vi "4Pi Capture Manager.vi"(7 "Calling VI Ref":refnum<vi>) -> ()   [LabVIEW 2016]
uses:
  4Pi Capture Manager Controls/4Pi Capture Switch Laser.ctl
  4Pi Capture Manager Controls/4Pi Capture Switch Line Scan Modes.ctl
  4Pi Capture Manager Controls/4Pi Capture Line Scan Settings.ctl
  4Pi Capture Manager Controls/DM scan mode.ctl
  <vilib>/Utility/miscctls.llb/LVPointTypeDef.ctl
  4Pi Capture Manager Controls/4Pi Capture Notifier Type.ctl
  4Pi Capture Manager Controls/4Pi Capture Actions.ctl
  4Pi Dual DM Control/4Pi Dual DM - Controls/4Pi Dual DM - Mirror Modes.ctl
  <vilib>/vision/Image Controls.llb/IMAQ Image.ctl
  Hardware Configuration/Hardware Configuration Controls/Device Type.ctl
  Hardware Configuration/Hardware Configuration Controls/Device Function.ctl
  Device Library/Cameras/Hamamatsu/Orca Flash/Orca Flash Controls/Orca Flash Actions.ctl
  Device Library/Cameras/Hamamatsu/Orca Flash/Orca Flash Controls/Orca Flash Parameters.ctl
  Device Library/Cameras/Hamamatsu/Orca Flash/Orca Flash Controls/Orca Flash Parameter List.ctl
  Device Library/Cameras/Hamamatsu/Orca Flash/Orca Flash Controls/Orca Flash ROI.ctl
  4Pi Capture Manager Controls/4Pi Capture Scan Tracker.ctl
  Device Manager/Common Device Queue/Common Device Controls/Common Device Actions.ctl
  Device Library/DAQmx/AO Single Channel Triggered Ramp/AO SCTR Type Defs/AO SCTR Actions.ctl
  Wide Field Drift Correction/WFDC Controls/WFDC External Sync.ctl
  Wide Field Drift Correction/WFDC Controls/WFDC Cycle Pause.ctl
  Wide Field Drift Correction/WFDC Controls/WFDC Status.ctl
  4Pi Dual DM Control/4Pi Dual DM - Controls/4Pi Dual DM - Standard Action.ctl
  Device Library/Stages/Stages Controls/Stage Actions.ctl
  Device Library/Shutters/Shutter Controls/Shutter Actions.ctl
  Device Library/AOTFs/AOTF Controls/AOTF Actions.ctl
  Device Library/Cameras/Camera Controls/Camera IMAQ Key Info.ctl
  Device Library/Cameras/Hamamatsu/Orca Flash/Orca Flash Controls/Orca Flash Notifier Element.ctl
  <vilib>/Utility/file.llb/Read Delimited Spreadsheet (DBL).vi
  <vilib>/Utility/file.llb/Write Delimited Spreadsheet (DBL).vi
  shell32.dll
panel:
  in  "Main Tab":T1(tab)
  in  "Sampling Time (s)":dbl min=0.0 format="%#_2f"
  out "Frame":u32(slide) scale=0.0..10.0
  out "Cycle":sgl(slide) scale=0.0..1.0
  in  "Base Save Path":path
  in  "Capture":bool
  in  "Live Preview":bool
  in  "Auto Shutter":bool=TRUE
  out "Z Step":sgl(slide) scale=0.0..1.0
  in  "File Name":string="Test Image"
  in  "Preview Exposure Time (s)":dbl=0.1 caption="Exposure Time (s)"
  in  "Capture Exposure Time (s)":dbl=0.1 caption="Exposure Time (s)"
  in  "No. of Frames":u32=1 min=1
  in  "No. of Cycles":u16=1 min=1
  in  "No. of Z Steps":u16=1 min=1
  in  "Z Step Size (µm)":dbl min=-10.0 max=10.0
  in  "Switch Laser At":T2=enum."Each Cycle"
  out "Current Cycle":u16
  out "Current Step":u16
  out "Current Frame":u32
  in  "Auto Update Subfolder":bool=TRUE
  in  "Subfolder Name":string="Area"
  in  "Current Laser":u16(ring) items=["560", "642", "405", "488", "940"]
  in  "Save As Preset":bool
  in  "Line Scan Active":bool
  in  "Number of Lines":u32=8 min=1 max=200 step=1
  in  "Line Scan Mode":T3
  in  "Line Scanning Presets":u16(ring) items=["01 FPS", "02 FPS", "04 FPS", "08 FPS", "16 FPS", "40 FPS"]
  in  "Line Scan Settings":T4
  in  "Soft trigger":bool
  in  "DM first":bool
  in  "Amp magnitude":dbl
  in  "DM scan mode":T5 items=["Idle", "Orthogonal", "Random"]
  in  "Amp step size":dbl
  in  "No. Amp steps":u16=1 min=1
  in  "Mirror Mode":u16[](array[numeric])=[1] min=1 max=140
  in  "Camera Settings":bool
  in  "Quadrants On/Off":bool
  in  "Quit":bool
  # "Live Preview"
  # "Capture"
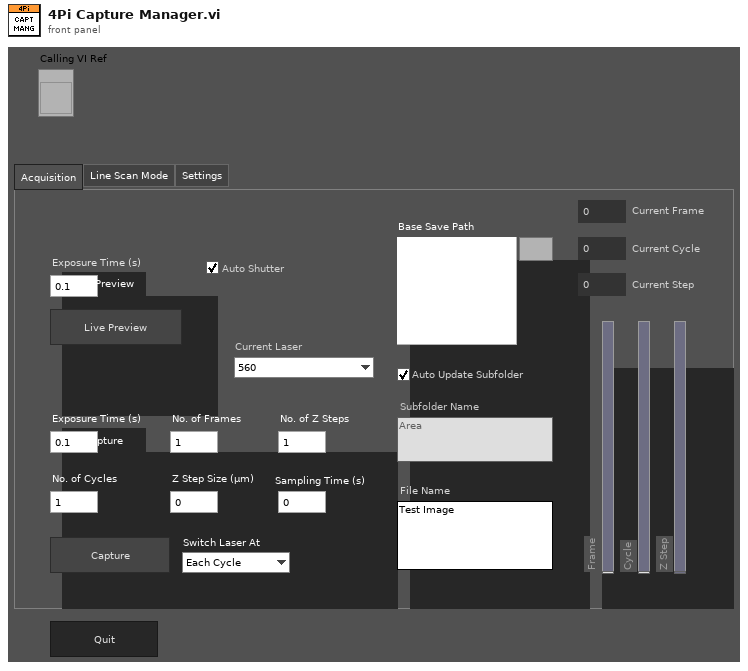
[diagram p1: front panel]
types:
  T1 = enum32{"Acquisition", "Line Scan Mode", "Settings"}
  T2 = typedef "4Pi Capture Switch Laser.ctl" = enum16{"Each Step", "Each Cycle", "All Cycles"}
  T3 = typedef "4Pi Capture Switch Line Scan Modes.ctl" = enum32{"Automatic", "Use Presets", "Manual"}
  T4 = typedef "4Pi Capture Line Scan Settings.ctl" = cluster{"Interline Interval":dbl, "Offset (V)":dbl, "Amplitude (V)":dbl, "Samples Per Channel":dbl, "Delay (ms)":dbl}
  T5 = typedef "DM scan mode.ctl" = u16
  T6 = typedef "IMAQ Image.ctl" = refnum<image>
  T7 = cluster{"Image Ref":T6, "Cycle Number":u16, "Camera Running?":bool, "Capture?":bool}
  T8 = enum8{"Enabled", "Disabled", "Disabled and Grayed Out"}
  T9 = typedef "Device Type.ctl" = enum16{"AOTF", "Camera", "Deformable Mirror", "Laser", "Flip Mirror", "Shutter", "Stage", "Waveform", "FPGA", "Email"}
  T10 = typedef "4Pi Capture Notifier Type.ctl" = cluster{"Actions":T11, "Running?":bool, "Preview Exposure (s)":dbl, "Capture Exposure (s)":dbl, "Cycles":u16, "Frames":u32, "No. of Z Steps":u16, "Z Step Size (µm)":dbl, "Base Path":path, "Init Z Position (µm)":dbl, "Lasers Lines":string[], "Save Path":path, "Line Scan?":bool, "Line Scan Mode":T3, "No. Amp steps":u16, "Amp step size":dbl, "No. Mirror Mode":u16, "DM scan mode":T5, "Metadata File Ref":refnum<file>[], "Init Mirror Modes":T12, "Sampling Time (s)":dbl}
  T11 = typedef "4Pi Capture Actions.ctl" = enum16{"Idle", "Live Preview", "Capture", "Laser On", "Laser Off", "Open Shutters", "Close Shutters", "Set Exposure Time", "Start Acquisition", "Update SubFolder", "Setup", "Camera Soft Trigger", "Camera", "Swtich1", "Switch", "Step", "Cycle", "Write DM", "External Cycle Sync", "Write Metadata", "Abort", "Quit"}
  T12 = typedef "4Pi Dual DM - Mirror Modes.ctl" = cluster{"Mode":string, "Amplitude":dbl}[]
  T13 = enum16{"Always On", "Always Off", "Off While Running"}
  T14 = typedef "LVPointTypeDef.ctl" = cluster{"Horizontal":i16, "Vertical":i16}
  T15 = typedef "Image Type" = u32
  T16 = typedef "Device Function.ctl" = enum16{"Primary", "Secondary", "Overview", "Wide Field Drift Correction", "642 nm Excitation", "560 nm Excitation", "940 nm Excitation", "546 nm Excitation", "488 nm Excitation", "405 nm Excitation", "Objective Drift Correction", "4Pi Focus Lock", "4Pi Objective Lock", "Objective XY", "Objective Z", "Sample XY", "Sample Coarse Z", "Sample Z", "4Pi Lower", "4Pi Upper", "Em Small", "Em Large", "Ex Small", "Ex Large", "Mojo", "Adj Cavity", "Line Scanning", "Alert"}
  T17 = typedef "Orca Flash Parameters.ctl" = cluster{"Value":dbl, "Parameter":T18}
  T18 = typedef "Orca Flash Parameter List.ctl" = u32
  T19 = enum32{"Page Enabled", "Page Disabled", "Page Disabled & Grayed"}
  T20 = typedef "Orca Flash ROI.ctl" = cluster{"H Offset":i32, "V Offset":i32, "H Width":i32, "V Width":i32}
  T21 = typedef "Orca Flash Actions.ctl" = enum16{"IDLE", "PREVIEW", "RECORD", "Send Trigger", "SOFT TRIGGER", "Record Settings", "SETPARAM", "GETPARAM", "SETROI", "GETROI", "PROGRESSIVE MODE", "AREA MODE", "STATUS", "QUIT"}
  T22 = typedef "4Pi Capture Scan Tracker.ctl" = cluster{"Current Step":u16, "Current Cycle":u16, "Current Laser":u16, "# of Lasers":u16, "# of Cycles":u16, "# of Steps":u16, "Switch Laser At":T2, "Current Mirror Mode":u16, "# of Mirror Mode":u16, "Current Amp step":u16, "# of Amp steps":u16}
  T23 = typedef "WFDC Status.ctl" = enum16{"Idle", "Busy", "DC Active", "Error"}
  T24 = typedef "WFDC External Sync.ctl" = cluster{"Cycle Sync":T25, "Z Offset":dbl, "WFDC Status":T23}
  T25 = typedef "WFDC Cycle Pause.ctl" = enum16{"Pause Requested", "Paused", "Resume Requested", "Resumed"}
  T26 = typedef "4Pi Dual DM - Standard Action.ctl" = enum16{"Read", "Write"}
  T27 = typedef "Stage Actions.ctl" = enum16{"Get Position", "SERVO OFF", "SERVO ON", "SERVO ON/OFF", "MVR", "MOVE", "HALT", "ONTARGET", "ERROR", "REFERENCE", "INIT", "VELOCITY", "STATUS", "EXIT", "HOME", "ZEROPOS", "NANOPOS", "ANALOG", "QUIT"}
  T28 = typedef "Shutter Actions.ctl" = enum16{"Open", "Close", "Toggle", "Status", "Quit"}
  T29 = typedef "AOTF Actions.ctl" = enum16{"Error Check", "Blank", "Line On/Off", "Set Power", "Status", "Quit"}
  T30 = typedef "AO SCTR Actions.ctl" = enum16{"Stop at Offset", "Update and Run", "Quit"}
  T31 = enum16{"open", "replace", "create", "open or create", "replace or create", "replace or create with confirmation"}
  T32 = typedef "Camera IMAQ Key Info.ctl" = cluster{"Frame":u32, "Sensor Height":i32, "Sensor Width":i32, "ROI Height":i32, "ROI Width":i32, "ROI Enable?":bool, "Bit per Pixel":u8}
  T33 = typedef "Orca Flash Notifier Element.ctl" = cluster{"Camera Actions":T21, "Received?":bool, "Running?":bool, "sCMOS Parameter":T17, "sCMOS ROI":T20, "Save Path":path, "# of frames":u32, "Image Ref":T6, "Trigger?":bool}
  T34 = typedef "Common Device Actions.ctl" = enum16{"Specific Action", "Open Front Panel", "Close Front Panel", "Quit", "Quit All"}
  T35 = typedef "4Pi Dual DM - Mirror Modes DUAL.ctl" = cluster{"Mode":string, "Amplitude":dbl}[][]
  T36 = typedef "LVRectTypeDef.ctl" = cluster{"Left":i16, "Top":i16, "Right":i16, "Bottom":i16}
  T37 = typedef "LVBoundsTypeDef.ctl" = cluster{"Width":u32, "Height":u32}
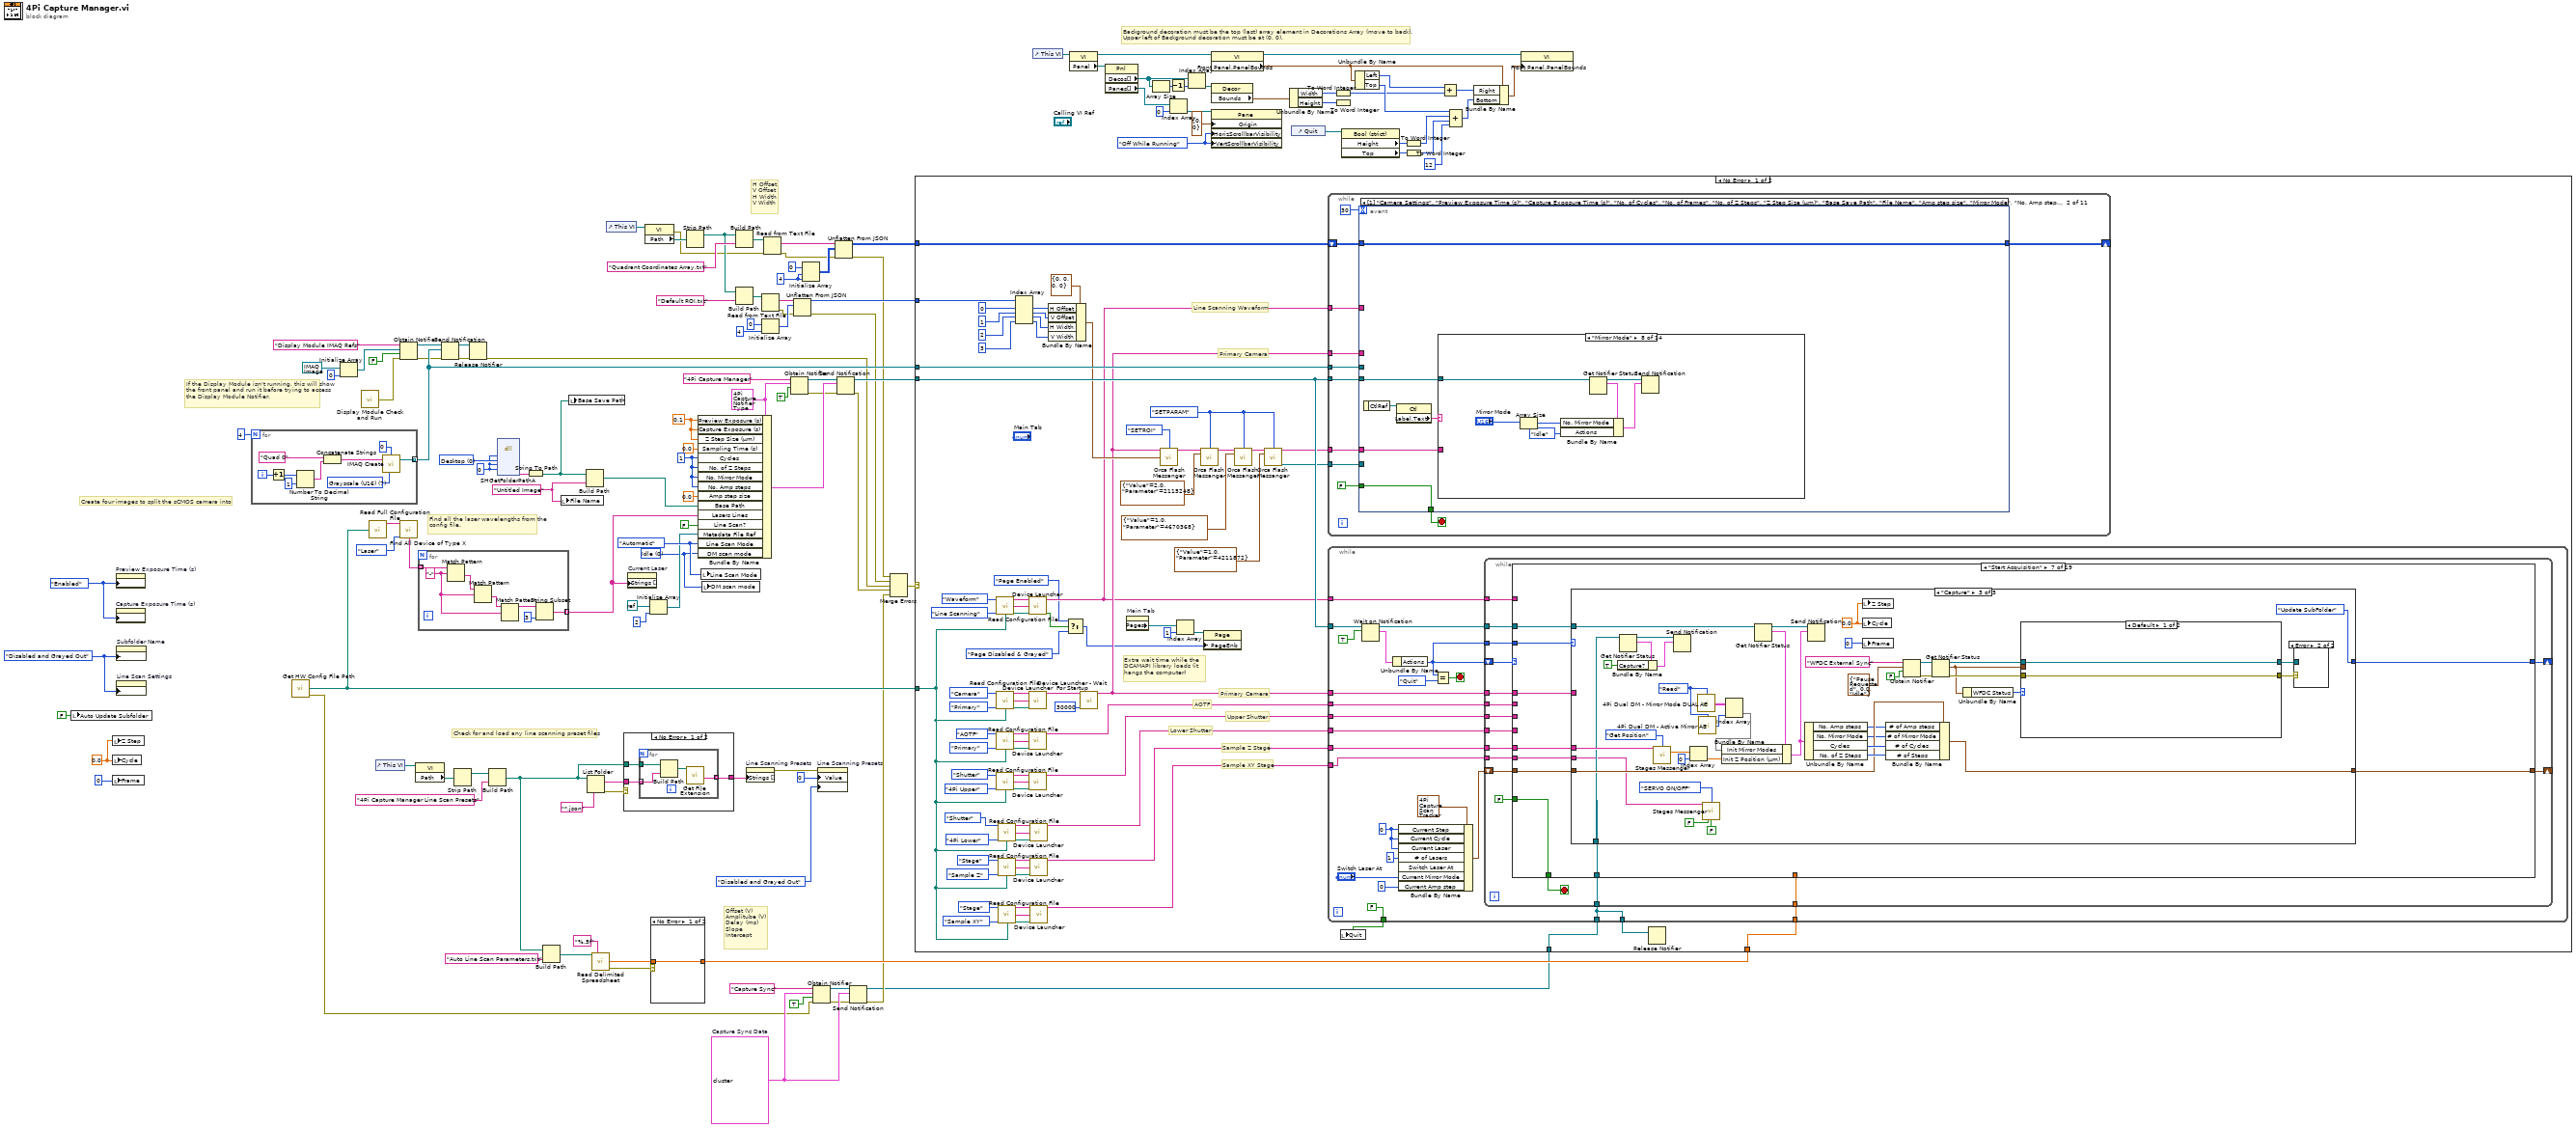
[diagram p0: block diagram]
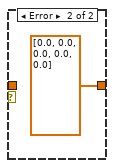
[diagram p2: hidden frame]
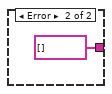
[diagram p3: hidden frame]
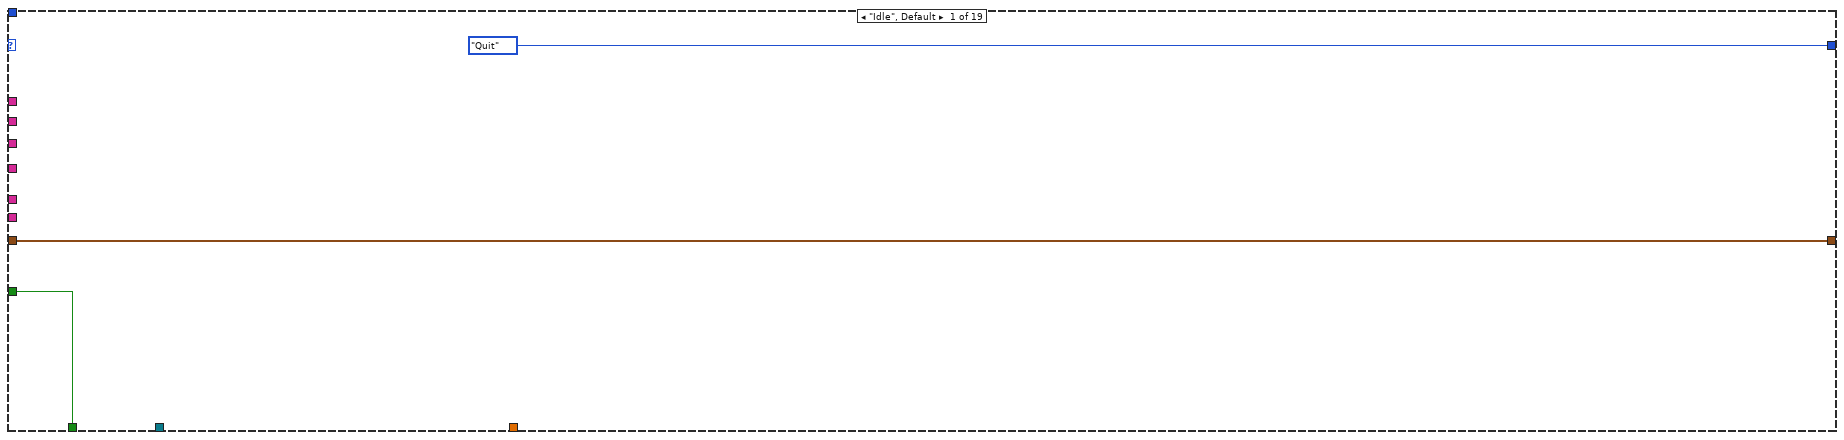
[diagram p4: hidden frame]
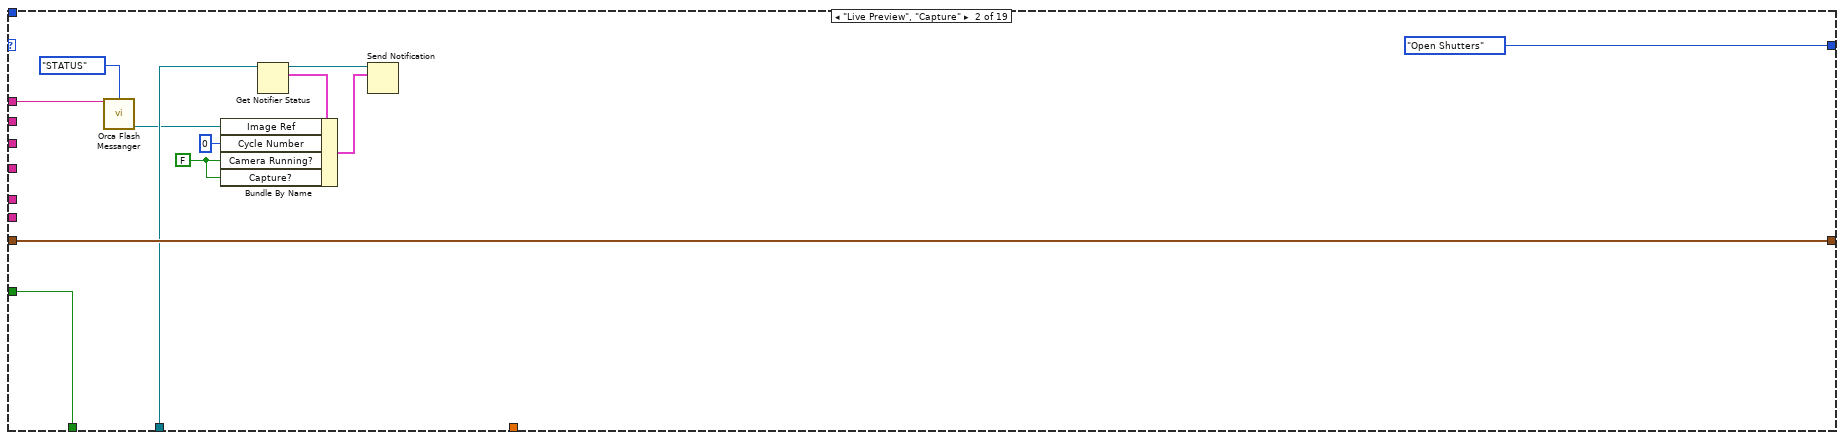
[diagram p5: hidden frame]
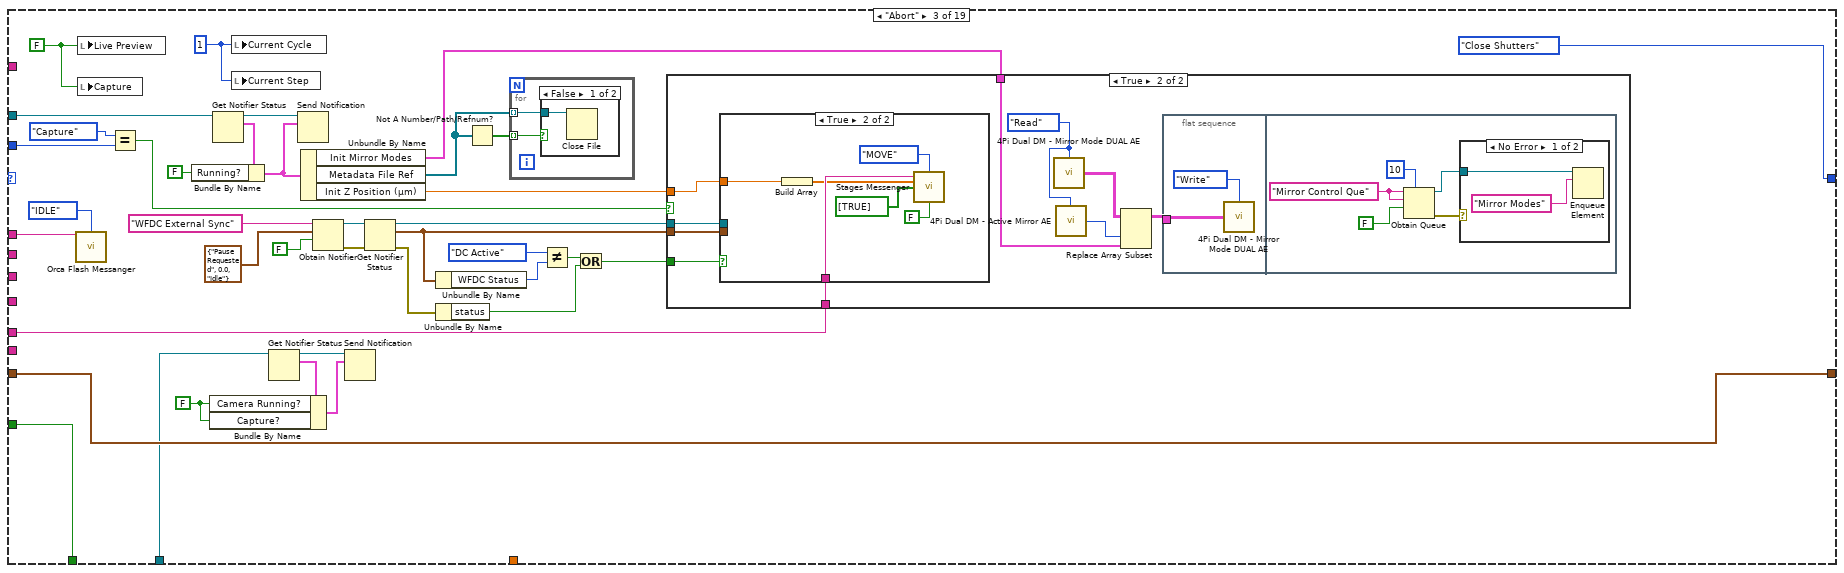
[diagram p6: hidden frame]
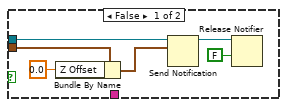
[diagram p10: hidden frame]
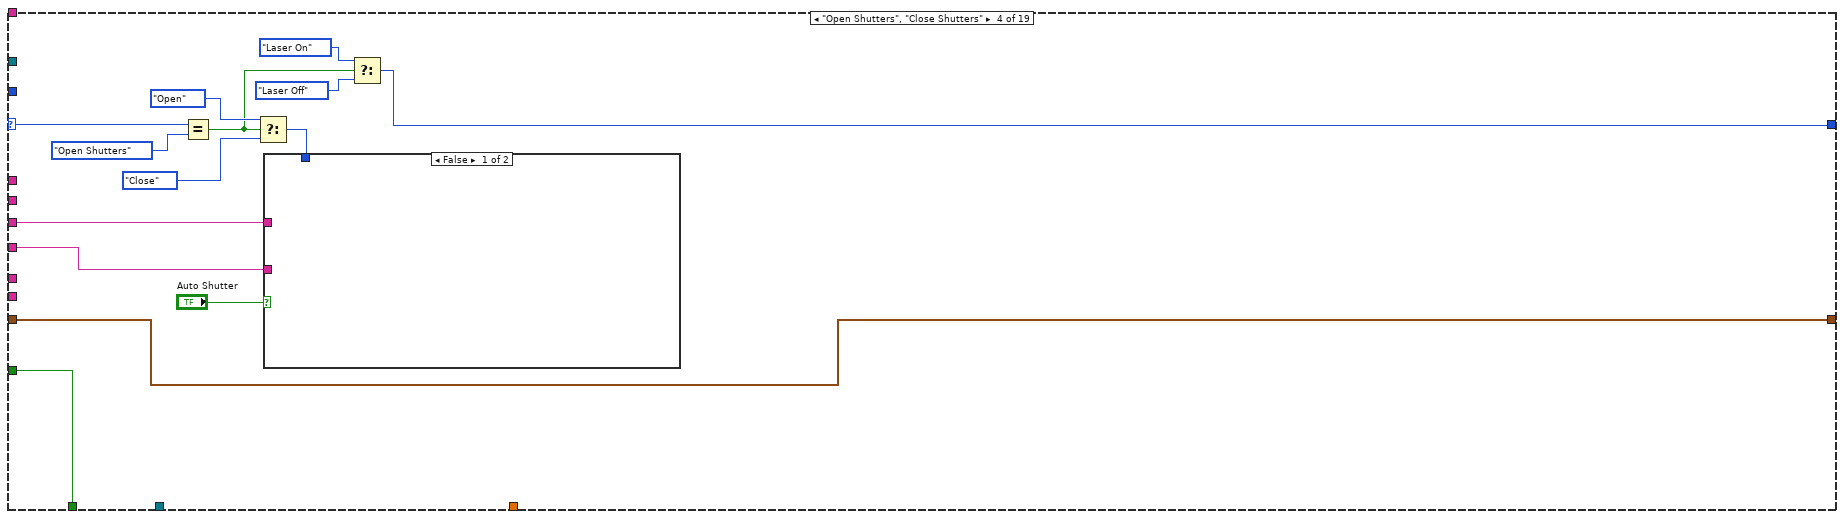
[diagram p11: hidden frame]
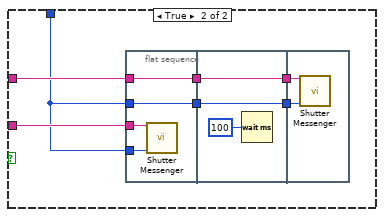
[diagram p12: hidden frame]
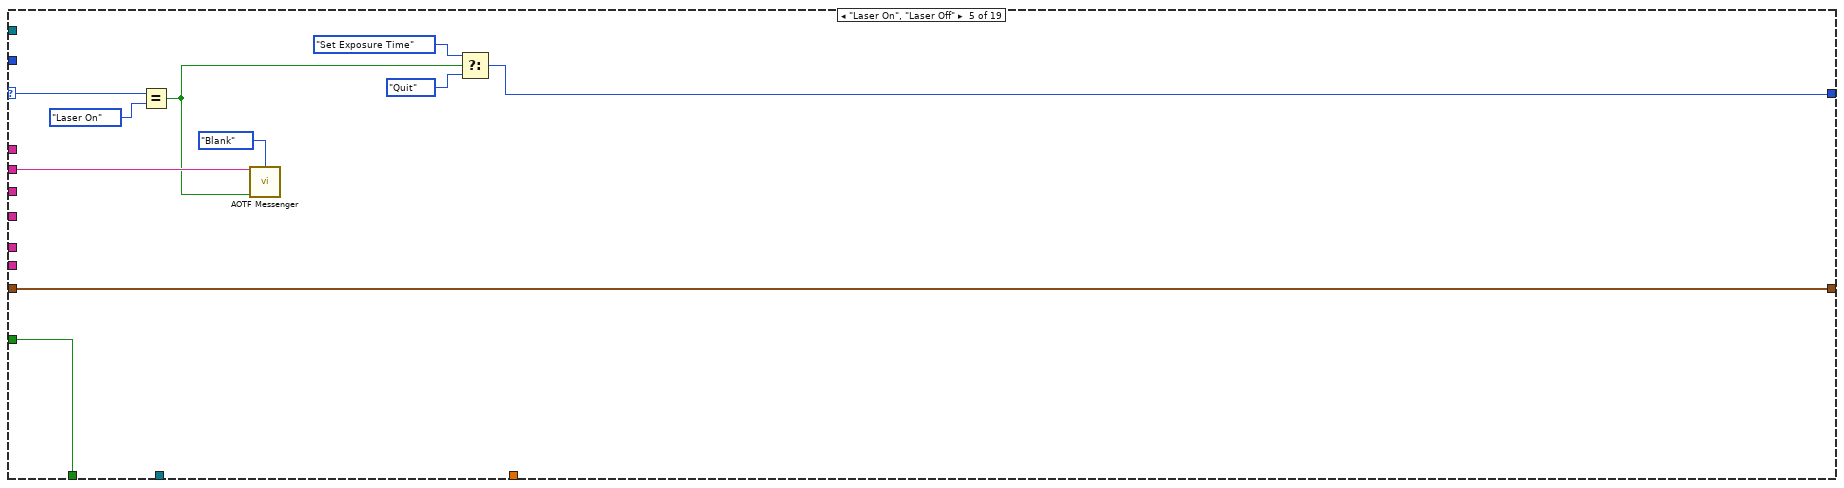
[diagram p13: hidden frame]
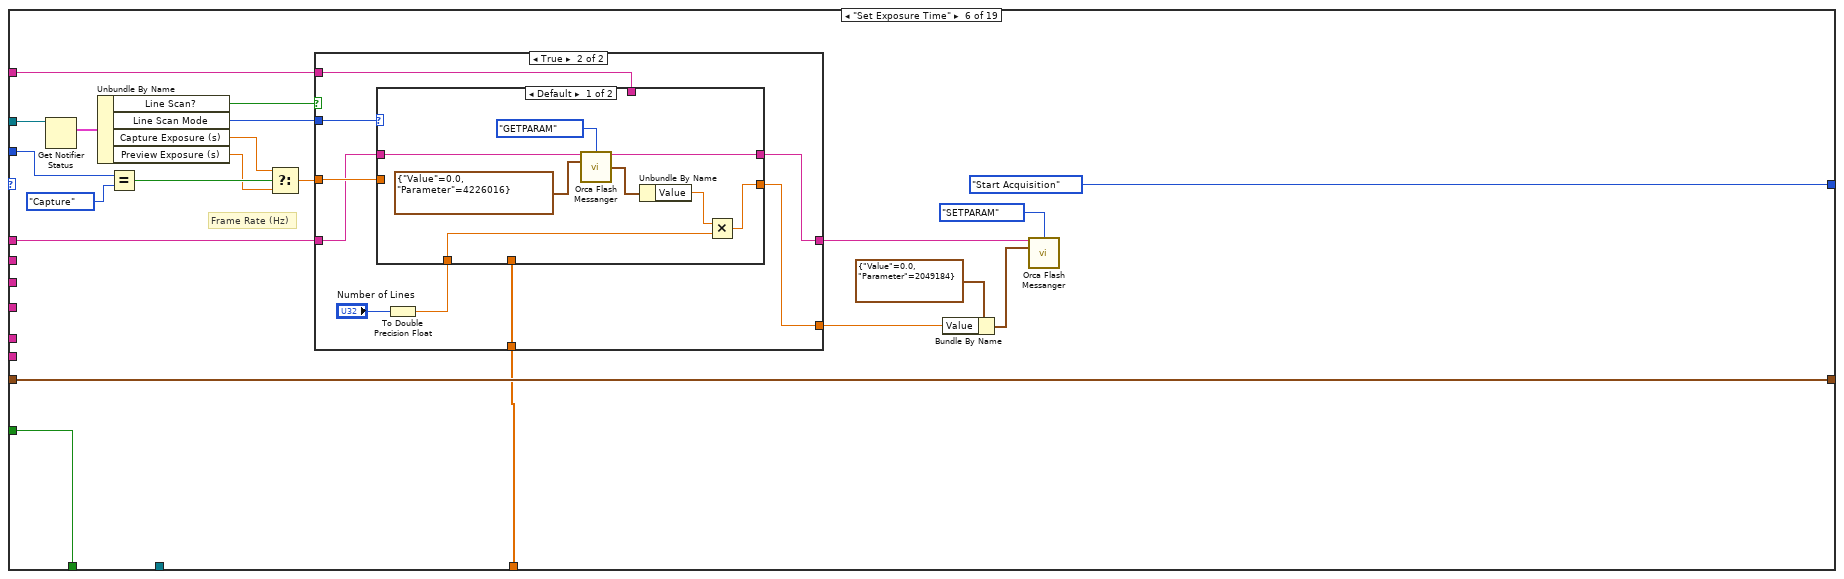
[diagram p14: hidden frame]
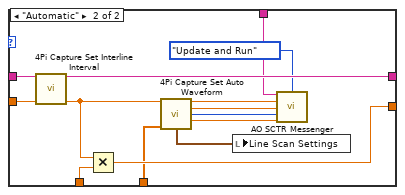
[diagram p16: hidden frame]
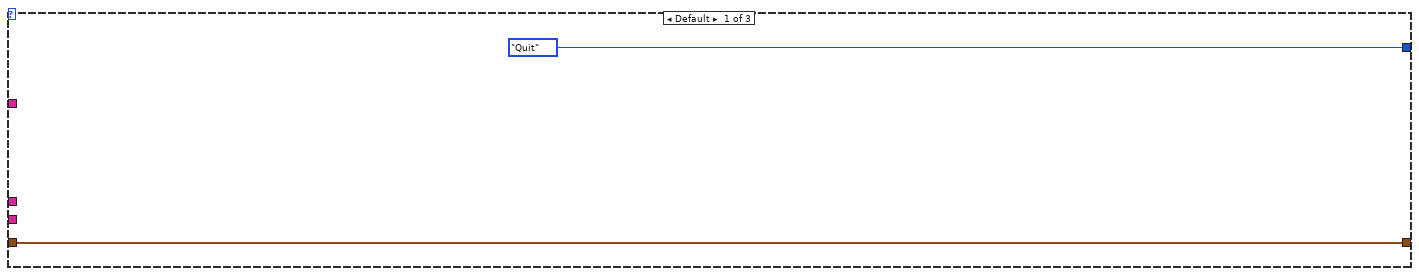
[diagram p17: hidden frame]
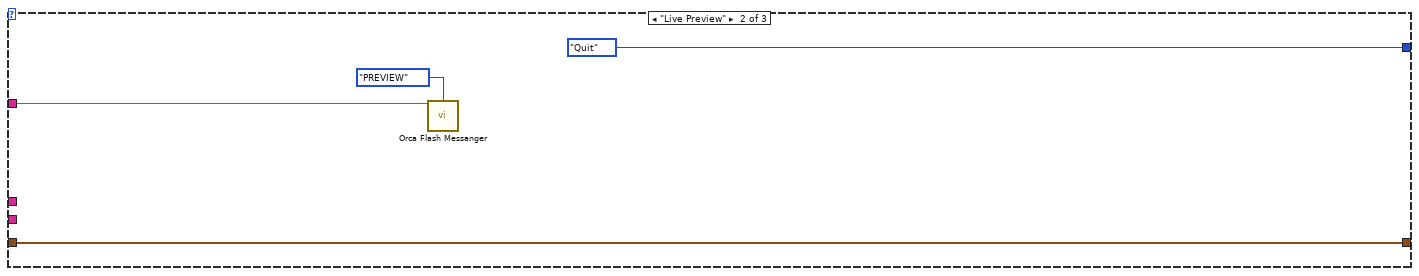
[diagram p18: hidden frame]
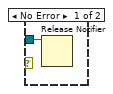
[diagram p19: hidden frame]
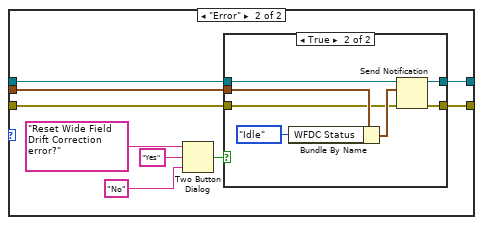
[diagram p20: hidden frame]
diagram:
  w5 = T5 0 items=["Idle", "Orthogonal", "Random"] ("DM scan mode")
  w15 = sgl 0.0 ("Cycle")
  w16 = T7 {"Image Ref"=refnum, "Cycle Number"=0, "Camera Running?"=FALSE, "Capture?"=FALSE}  # Capture Sync Data
  w28 = T8."Enabled" ("Disabled")
  w9 = 4Pi_Capture_Switch_Line_Scan_Modes."Automatic" ("Line Scan Mode")
  w29 = T8."Disabled and Grayed Out" ("Disabled")
  w76 = 4 ("dimension size")
  w80 = "Untitled Image"
  w83 = 0 items=["Desktop"=0, "Personal Documents"=5, "AppData"=26, "Local AppData"=28, "Common AppData"=35, "Program Files"=38, "Program Files Common"=43, "Common Documents"=46] ("Requested Path")
  w82 = 0 ("HWND")
  w4 = u16 1 ("Cycles")
  w3 = 0.1 ("Preview Exposure (s)")
  w86 = T10 {"Actions"=enum."Live Preview", "Running?"=FALSE, "Preview Exposure (s)"=0.1, "Capture Exposure (s)"=0.1, "Cycles"=1, "Frames"=0, "No. of Z Steps"=0, "Z Step Size (µm)"=0.0, "Base Path"=path "", "Init Z Position (µm)"=0.0, "Lasers Lines"=[], "Save Path"=path "", "Line Scan?"=FALSE, "Line Scan Mode"=enum."Automatic", "No. Amp steps"=0, "Amp step size"=0.0, "No. Mirror Mode"=0, "DM scan mode"=0, "Metadata File Ref"=[], "Init Mirror Modes"=[], "Sampling Time (s)"=0.0} ("4Pi Capture Notifier Type")
  w108 = T13."Off While Running" ("Vertical Scrollbar Visibility")
  # "Offset (V)\nAmplitube (V)\nDelay (ms)\nSlope\nIntercept"
  # "Check for and load any line scanning preset files"
  # "Find all the laser wavelengths from the config file."
  # "If the Display Module isn't running, this will show the front panel and run it before trying to access the Display Module Notifier."
  # "H Offset\nV Offset\nH Width\nV Width"
  # "Create four images to split the sCMOS camera into"
  # "Background decoration must be the top (last) array element in Decorations Array (move to back).\nUpper left of Background decoration must be at (0, 0)."
  n1 = local write "Auto Update Subfolder"(FALSE ("Auto Update Subfolder")) -> ()
  n2 = local write "Z Step"(w15) -> ()
  n3 = local write "Cycle"(w15) -> ()
  n4 = local write "Frame"(u32 0 ("Frame")) -> ()
  n5 = property on="Preview Exposure Time (s)" class="DigNum (strict)"("DisabledEnum"=w28) -> ()  [unwired: 2 in, 2 out]
  n6 = property on="Capture Exposure Time (s)" class="DigNum (strict)"("DisabledEnum"=w28) -> ()  [unwired: 2 in, 2 out]
  n7 = property on="Subfolder Name" class="Str"("DisabledEnum"=w29) -> ()  [unwired: 2 in, 2 out]
  n8 = property on="Line Scan Settings" class="Clust (strict)"("DisabledEnum"=w29) -> ()  [unwired: 2 in, 2 out]
  n9 = for {
    N: 4 -> [_]
    tunnel: [w126] -> w90 mode=indexing
    i -> [w134]
    w129 = T15 7 items=["Grayscale (U8)", "Grayscale (I16)", "Grayscale (SGL)", "Complex (CSG)", "RGB (U32)", "HSL (U32)", "RGB (U64)", "Grayscale (U16)"] ("Image Type")
    n10 = Increment(x=w134) -> (x+1=w132:i32)
    n11 = Number To Decimal String(number=w132, width (-)=i16 1) -> (decimal integer string=w130:string)
    n12 = Concatenate Strings("Quad 0" ("name (unnamed)"), w130) -> (w127:string)
    n13 = call "IMAQ Create"("Border Size"=0, "Image Name"=w127, "Image Type"=w129) -> ("New Image"=w126:T6)  [unwired: 2 in, 1 out]
  }
  n14 = call "Get HW Config File Path.vi"() -> ("File Path"=w43:path, "Error"=w13:errorcluster)  [unwired: 14 in]
  n15 = Initialize Array(T6 refnum ("New Image"), 0 ("dimension size")) -> (w48:T6[])
  n16 = call "Display Module Check and Run.vi"() -> ("Error"=w47:errorcluster)  [unwired: 15 in]
  n17 = call "Read Full Configuration File.vi"("Config File Path"=w43) -> ("Unique Notifier Names"=w44:string[])  [unwired: 11 in, 3 out]
  n18 = control-ref of="This VI"() -> (w40:refnum<vi>)
  n19 = Obtain Notifier(name (unnamed)="Display Module IMAQ Refs", notification data type=w48, create if not found? (T)=FALSE, error in (no error)=w47) -> (notifier out=w91:refnum<notifier>, error out=w58:errorcluster)  [unwired: 1 out]
  n20 = call "Find All Device of Type X.vi"("Unique Notifier Names"=w44, "Device Type"=Device_Type."Laser") -> ("All Devices"=w46:string[])  [unwired: 12 in, 1 out]
  n21 = property class="VI"(reference=w40) -> ("Path"=w39:path)  [unwired: 1 in, 2 out]
  n22 = for {
    tunnel: w46 -> [w136] mode=indexing
    tunnel: [w135] -> w20 mode=indexing
    w139 = "-" ("regular expression")
    n23 = Match Pattern(string=w136, regular expression=w139) -> (after substring=w137:string)  [unwired: 1 in, 3 out]
    n24 = Match Pattern(string=w137, regular expression=w139) -> (after substring=w138:string)  [unwired: 1 in, 3 out]
    n25 = Match Pattern(string=w138, regular expression=w139) -> (before substring=w140:string)  [unwired: 1 in, 3 out]
    n26 = String Subset(string=w140, length (rest)=3 ("length (rest)")) -> (substring=w135:string)  [unwired: 1 in]
  }
  n27 = Send Notification(notification=w90, notifier=w91, error in (no error)=w58) -> (notifier out=w78:refnum<notifier>, error out=w63:errorcluster)
  n28 = Strip Path(path=w39) -> (stripped path=w38:path)  [unwired: 1 out]
  n29 = Release Notifier(notifier=w78, error in (no error)=w63) -> (error out=w55:errorcluster)  [unwired: 1 in, 2 out]
  n30 = Build Path(base path=w38, name or relative path="4Pi Capture Manager Line Scan Presets") -> (appended path=w27:path)
  n31 = dll-call lib="shell32.dll" fn="SHGetFolderPathA"("HWND"=w82, "nFolder"=w83, "hToken"=w82, "dwFlags"=w82) -> ("pszPath"=w81:string)  [unwired: 9 in, 2 out]
  n32 = String To Path(string=w81) -> (path=w79:path)
  n33 = Build Path(base path=w27, name or relative path="Auto Line Scan Parameters.txt") -> (appended path=w25:path)
  n34 = local write "File Name"(w80) -> ()
  n35 = local write "Base Save Path"(w79) -> ()
  n36 = Build Path(base path=w79, name or relative path=w80) -> (appended path=w84:path)
  n37 = List Folder(path=w27, pattern="*.json") -> (filenames=w35:string[], error out=w34:errorcluster)  [unwired: 2 in, 2 out]
  n38 = call-poly <vilib>:"Read Delimited Spreadsheet.vi"("file path (dialog if empty)"=w25, "format (%.3f)"="%.5f") -> ("first row"=w22:dbl[], "error out"=w23:errorcluster)  [unwired: 8 in, 4 out]
  n39 = control-ref of="This VI"() -> (w89:refnum<vi>)
  n40 = case shown="No Error" w34 {
    tunnel: w35 -> [w144 _]
    tunnel: w27 -> [w143 _]
    tunnel: [w142 string[] []] -> w33
    frame No Error {
      n41 = for {
        tunnel: w144 -> [w147] mode=indexing
        tunnel: w143 -> [w148]
        tunnel: [w145] -> w142 mode=indexing
        n42 = Build Path(base path=w148, name or relative path=w147) -> (appended path=w146:path)
        n43 = call <vilib>:"Get File Extension.vi"("file"=w146) -> ("filename without extension"=w145:string)  [unwired: 6 in, 4 out]
      }
    }
    frame Error {
    }
  }
  n44 = property on="Current Laser" class="Ring (strict)"("Strings []"=w20) -> ()  [unwired: 2 in, 2 out]
  n45 = property class="VI"(reference=w89) -> (error out=w60:errorcluster, "Path"=w88:path)  [unwired: 1 in, 1 out]
  n46 = Initialize Array(refnum<k0> refnum, 2 ("dimension size")) -> (w6:refnum<k0>[])
  n47 = case shown="No Error" w23 {
    tunnel: w22 -> [w150 _]
    tunnel: [w150 dbl[] [0.0, 0.0, 0.0, 0.0, 0.0] ("first row")] -> w21
    frame No Error {
    }
    frame Error {
    }
  }
  n48 = Strip Path(path=w88) -> (stripped path=w71:path)  [unwired: 1 out]
  n49 = Bundle By Name(cluster=w86, "Preview Exposure (s)"=w3, "Capture Exposure (s)"=w3, "Z Step Size (µm)"=w3, "Sampling Time (s)"=0.0, "Cycles"=w4, "No. of Z Steps"=w4, "No. Mirror Mode"=w4, "No. Amp steps"=w4, "Amp step size"=0.0, "Base Path"=w84, "Lasers Lines"=w20, "Line Scan?"=FALSE, "Metadata File Ref"=w6, "Line Scan Mode"=w9, "DM scan mode"=w5) -> (w85:T10)
  n50 = local write "Line Scan Mode"(w9) -> ()
  n51 = local write "DM scan mode"(w5) -> ()
  n52 = Build Path(base path=w71, name or relative path="Quadrant Coordinates Array.txt") -> (appended path=w74:path)
  n53 = Build Path(base path=w71, name or relative path="Default ROI.txt") -> (appended path=w69:path)
  n54 = property on="Line Scanning Presets" class="Ring (strict)"("Strings []"=w33) -> (error out=w32:errorcluster)  [unwired: 2 in, 1 out]
  n55 = Read from Text File(file (use dialog)=w69) -> (text=w68:string, error out=w61:errorcluster)  [unwired: 3 in, 2 out]
  n56 = Initialize Array(0 ("element"), 4 ("dimension size")) -> (w65:i32[])
  n57 = Read from Text File(file (use dialog)=w74, error in=w60) -> (text=w73:string, error out=w59:errorcluster)  [unwired: 2 in, 2 out]
  n58 = Obtain Notifier(name (unnamed)="4Pi Capture Manager", notification data type=w86, create if not found? (T)=TRUE) -> (notifier out=w94:refnum<notifier>, error out=w62:errorcluster)  [unwired: 1 in, 1 out]
  n59 = Unflatten From JSON(JSON string=w68, type and defaults=w65, error in (no error)=w61) -> (value=w64:i32[], error out=w54:errorcluster)  [unwired: 4 in]
  n60 = Initialize Array(0 ("element"), w76, w76) -> (w75:i32[][])
  n61 = Obtain Notifier(name (unnamed)="Capture Sync", notification data type=w16, create if not found? (T)=TRUE, error in (no error)=w13) -> (notifier out=w17:refnum<notifier>, error out=w12:errorcluster)  [unwired: 1 out]
  n62 = property on="Line Scanning Presets" class="Ring (strict)"(error in=w32, "Value"=u16 0, "DisabledEnum"=T8."Disabled and Grayed Out" ("Disabled")) -> ()  [unwired: 1 in, 2 out]
  n63 = Unflatten From JSON(JSON string=w73, type and defaults=w75, error in (no error)=w59) -> (value=w72:i32[][], error out=w53:errorcluster)  [unwired: 4 in]
  n64 = Send Notification(notification=w85, notifier=w94, error in (no error)=w62) -> (notifier out=w93:refnum<notifier>, error out=w56:errorcluster)
  n65 = Send Notification(notification=w16, notifier=w17, error in (no error)=w12) -> (notifier out=w10:refnum<notifier>, error out=w11:errorcluster)
  n66 = Merge Errors(w53, w54, w55, w56, w11) -> (w57:errorcluster)
  n67 = case shown="No Error" w57 {
    tunnel: w43 -> [w153 _]
    tunnel: w93 -> [w211 w1561]
    tunnel: w90 -> [w199 w1559]
    tunnel: w72 -> [w198 _]
    tunnel: w64 -> [w192 _]
    tunnel: w21 -> [w173 _]
    tunnel: w10 -> [w165 _]
    frame No Error {
      w159 = Orca_Flash_Actions."SETPARAM" ("Camera Actions")
      # "Sample XY Stage"
      # "Line Scanning Waveform"
      # "Primary Camera"
      # "Extra wait time while the DCAMAPI library loads (it hangs the computer)"
      # "Sample Z Stage"
      # "Lower Shutter"
      # "Upper Shutter"
      # "AOTF"
      # "Primary Camera"
      n68 = call "Read Configuration File.vi"("Device Type"=Device_Type."Waveform", "Device Function"=Device_Function."Line Scanning", "Config File Path"=w153) -> ("Unique Notifier Name"=w177:string, "Device Ports/IDs/Channels"=w178:string[], "Device Engine Path"=w175:path)  [unwired: 9 in, 1 out]
      n69 = call "Read Configuration File.vi"("Device Type"=Device_Type."Camera", "Device Function"=Device_Function."Primary", "Config File Path"=w153) -> ("Unique Notifier Name"=w231:string, "Device Ports/IDs/Channels"=w230:string[], "Device Engine Path"=w229:path)  [unwired: 9 in, 1 out]
      n70 = call "Read Configuration File.vi"("Device Type"=Device_Type."AOTF", "Device Function"=Device_Function."Primary", "Config File Path"=w153) -> ("Unique Notifier Name"=w222:string, "Device Ports/IDs/Channels"=w223:string[], "Device Engine Path"=w224:path)  [unwired: 9 in, 1 out]
      n71 = call "Read Configuration File.vi"("Device Type"=Device_Type."Shutter", "Device Function"=Device_Function."4Pi Upper", "Config File Path"=w153) -> ("Unique Notifier Name"=w212:string, "Device Ports/IDs/Channels"=w221:string[], "Device Engine Path"=w220:path)  [unwired: 9 in, 1 out]
      n72 = call "Read Configuration File.vi"("Device Type"=Device_Type."Shutter", "Device Function"=Device_Function."4Pi Lower", "Config File Path"=w153) -> ("Unique Notifier Name"=w213:string, "Device Ports/IDs/Channels"=w216:string[], "Device Engine Path"=w217:path)  [unwired: 9 in, 1 out]
      n73 = call "Read Configuration File.vi"("Device Type"=Device_Type."Stage", "Device Function"=Device_Function."Sample Z", "Config File Path"=w153) -> ("Unique Notifier Name"=w206:string, "Device Ports/IDs/Channels"=w204:string[], "Device Engine Path"=w203:path)  [unwired: 9 in, 1 out]
      n74 = call "Read Configuration File.vi"("Device Type"=Device_Type."Stage", "Device Function"=Device_Function."Sample XY", "Config File Path"=w153) -> ("Unique Notifier Name"=w154:string, "Device Ports/IDs/Channels"=w158:string[], "Device Engine Path"=w157:path)  [unwired: 9 in, 1 out]
      n75 = Index Array(array=w192, index #1=0 ("index"), index #2=1 ("index"), index #3=2 ("index"), index #4=3 ("index")) -> (element #1=w187:i32, element #2=w184:i32, element #3=w185:i32, element #4=w186:i32)
      n76 = call "Device Launcher.vi"("Notifier Name"=w177, "Device Ports/IDs/Channels"=w178, "Device Engine Path"=w175) -> ("Notifier Name"=w174:string, "Running?"=w169:bool)  [unwired: 11 in]
      n77 = call "Device Launcher.vi"("Notifier Name"=w231, "Device Ports/IDs/Channels"=w230, "Device Engine Path"=w229) -> ("Notifier Name"=w181:string)  [unwired: 11 in, 1 out]
      n78 = call "Device Launcher.vi"("Notifier Name"=w222, "Device Ports/IDs/Channels"=w223, "Device Engine Path"=w224) -> ("Notifier Name"=w210:string)  [unwired: 11 in, 1 out]
      n79 = call "Device Launcher.vi"("Notifier Name"=w212, "Device Ports/IDs/Channels"=w221, "Device Engine Path"=w220) -> ("Notifier Name"=w209:string)  [unwired: 11 in, 1 out]
      n80 = call "Device Launcher.vi"("Notifier Name"=w213, "Device Ports/IDs/Channels"=w216, "Device Engine Path"=w217) -> ("Notifier Name"=w208:string)  [unwired: 11 in, 1 out]
      n81 = call "Device Launcher.vi"("Notifier Name"=w206, "Device Ports/IDs/Channels"=w204, "Device Engine Path"=w203) -> ("Notifier Name"=w201:string)  [unwired: 11 in, 1 out]
      n82 = call "Device Launcher.vi"("Notifier Name"=w154, "Device Ports/IDs/Channels"=w158, "Device Engine Path"=w157) -> ("Notifier Name"=w152:string)  [unwired: 11 in, 1 out]
      n83 = Bundle By Name(cluster=T20 {"H Offset"=0, "V Offset"=0, "H Width"=0, "V Width"=0} ("Orca Flash ROI"), "H Offset"=w187, "V Offset"=w184, "H Width"=w185, "V Width"=w186) -> (w183:T20)
      n84 = Select(t=T19."Page Enabled" ("Page Enabled State"), s=w169, f=T19."Page Disabled & Grayed" ("Page Enabled State")) -> (s? t:f=w166:T19)
      n85 = call "Device Launcher - Wait For Startup.vi"("Notifier Name"=w181, "Wait Time (ms)"=30000) -> ("Notifier Name (Dup)"=w180:string)  [unwired: 12 in, 1 out]
      n86 = property on="Main Tab" class="TabCtl (strict)"() -> ("Pages"=w172:refnum<vi>[])  [unwired: 2 in, 2 out]
      n87 = call "Orca Flash Messanger.vi"("Notifier Name"=w180, "Camera Actions"=Orca_Flash_Actions."SETROI", "sCMOS ROI"=w183) -> ("Notifier Name Dup"=w197:string)  [unwired: 8 in, 4 out]
      n88 = Index Array(array=w172, index=1) -> (element=w170:refnum<vi>)
      n89 = call "Orca Flash Messanger.vi"("Notifier Name"=w197, "Camera Actions"=w159, "sCMOS Parameter"=T17 {"Value"=2.0, "Parameter"=2115248}) -> ("Notifier Name Dup"=w196:string)  [unwired: 8 in, 4 out]
      n90 = property class="Page"(reference=w170, "PageEnb"=w166) -> ()  [unwired: 1 in, 2 out]
      n91 = call "Orca Flash Messanger.vi"("Notifier Name"=w196, "Camera Actions"=w159, "sCMOS Parameter"=T17 {"Value"=1.0, "Parameter"=4670368}) -> ("Notifier Name Dup"=w163:string)  [unwired: 8 in, 4 out]
      n92 = call "Orca Flash Messanger.vi"("Notifier Name"=w163, "Camera Actions"=w159, "sCMOS Parameter"=T17 {"Value"=1.0, "Parameter"=4211872}) -> ("Notifier Name Dup"=w162:string, "Image Ref"=w161:T6)  [unwired: 8 in, 3 out]
      n93 = while {
        tunnel: w211 -> [w1161]
        tunnel: w162 -> [w1160]
        tunnel: w161 -> [w1158]
        tunnel: w199 -> [w1157]
        shift-right: [w1155] -> _
        shift-left: w198 -> [w1156]
        tunnel: w180 -> [w1154]
        tunnel: w174 -> [w1153]
        stop <- w1163 stop-if-true
        n94 = event shown="[1] \"Camera Settings\", \"Preview Exposure Time (s)\", \"Capture Exposure Time (s)\", \"No. of Cycles\", \"No. of Frames\", \"No. of Z Steps\", \"Z Step Size (µm)\", \"Base Save Path\", \"File Name\", \"Amp step size\", \"Mirror Mode\", \"No. Amp steps\", \"DM scan mode\", \"Sampling Time (s)\": Value Change" {
          selector: _ -> [_ _ _ _ _ _ _ _ _ _ _]
          dyn-events: _ -> [_ _ _ _ _ _ _ _ _ _ _]
          timeout: 30 -> [_ _ _ _ _ _ _ _ _ _ _]
          tunnel: [w1187 w1225 w1344 w1365 w1421 w1446 w1468 w1484 w1504 w1528 w1557] -> w1163
          tunnel: FALSE -> [w1187 w1225 w1344 w1365 w1421 w1446 w1468 w1484 w1504 w1528 _]
          tunnel: w1161 -> [w1181 w1222 w1341 _ _ w1440 w1466 _ w1502 _ w1556]
          tunnel: w1160 -> [_ w1221 _ _ _ _ _ _ _ _ _]
          tunnel: w1158 -> [w1185 _ _ w1349 _ _ _ _ _ _ _]
          tunnel: w1157 -> [w1186 _ _ w1355 _ _ _ _ _ _ w1544]
          tunnel: w1156 -> [w1184 w1220 w1333 w1348 w1416 w1423 w1467 w1485 w1503 w1520 w1543]
          tunnel: [w1184 w1220 w1333 w1347 w1416 w1423 w1467 w1485 w1503 w1520 w1543] -> w1155
          tunnel: w1154 -> [_ _ _ _ _ w1434 _ _ w1488 _ _]
          tunnel: w1153 -> [_ _ _ _ _ w1424 _ _ w1496 _ _]
          event Timeout {
            # "Convert to array and then crop. If you\nextract or mask image the destination\nimage custom data keys are overwritten."
            n95 = event-data() -> ()  [unwired: 1 in, 1 out]
            n96 = call "IMAQ ImageToArray"("Image"=w1185) -> ("Image Pixels (U16)"=w1183:u16[][])  [unwired: 3 in, 4 out]
            n97 = for {
              tunnel: w1186 -> [w1218] mode=indexing
              tunnel: w1183 -> [w1219]
              tunnel: w1184 -> [w1216] mode=indexing
              n98 = Index Array(array=w1216, index #1=0 ("index"), index #2=2 ("index"), index #3=1 ("index"), index #4=3 ("index")) -> (element #1=w1214:i32, element #2=w1213:i32, element #3=w1209:i32, element #4=w1208:i32)
              n99 = Array Subset(array=w1219, index (row)=w1214, length (row)=w1213, index (col)=w1209, length (col)=w1208) -> (w1217:u16[][])
              n100 = call "IMAQ ArrayToImage"("Image Pixels (U16)"=w1217, "Image"=w1218) -> ()  [unwired: 8 in, 2 out]
            }
            n101 = local read "Soft trigger"() -> (w1166:bool)
            n102 = local read "No. Amp steps"() -> (w1165:u16)
            n103 = case shown="True" w1166 {
              tunnel: [w1188 w1189] -> w1164
              tunnel: w1165 -> [_ w1190]
              frame False {
                n104 = local read "No. of Frames"() -> (w1188:u32)
              }
              frame True {
                n105 = To Unsigned Long Integer(number=w1190) -> (unsigned 32bit integer=w1189:u32)
                n106 = local write "No. of Frames"(w1189) -> ()
              }
            }
            n107 = local read "Mirror Mode"() -> (w1175:u16[])
            n108 = local read "Soft trigger"() -> (w1168:bool)
            n109 = local read "DM scan mode"() -> (w1173:T5)
            n110 = local read "No. of Cycles"() -> (w1171:u16)
            n111 = local read "Amp step size"() -> (w1176:dbl)
            n112 = local read "DM first"() -> (w1169:bool)
            n113 = local read "Z Step Size (µm)"() -> (w1177:dbl)
            n114 = local read "No. of Z Steps"() -> (w1178:u16)
            n115 = Array Size(array=w1175) -> (size(s)=w1172:i32)
            n116 = Or(x=w1169, y=w1168) -> (x .or. y?=w1167:bool)
            n117 = case shown="1" w1173 {
              tunnel: w1172 -> [_ w1195]
              tunnel: w1165 -> [_ w1196]
              tunnel: [w1191 w1194] -> w1170
              tunnel: w1167 -> [_ w1193]
              tunnel: w1171 -> [w1191 w1192]
              frame Default {
              }
              frame 1 {
                n118 = case shown="True" w1193 {
                  tunnel: w1196 -> [w1202 _]
                  tunnel: w1195 -> [w1201 w1207]
                  tunnel: [w1197 w1206] -> w1194
                  tunnel: w1192 -> [_ _]
                  frame False {
                    n119 = To Unsigned Word Integer(number=w1201) -> (unsigned 16bit integer=w1200:u16)
                    n120 = Multiply(x=w1200, y=w1202) -> (x*y=w1198:u16)
                    n121 = Equal To 0?(x=w1198) -> (x = 0?=w1199:bool)
                    n122 = case shown="False" w1199 {
                      tunnel: w1198 -> [w1203 w1205]
                      tunnel: [w1203 w1204] -> w1197
                      frame False {
                      }
                      frame True {
                        n123 = Increment(x=w1205) -> (x+1=w1204:u16)
                      }
                    }
                  }
                  frame True {
                    n124 = To Unsigned Word Integer(number=w1207) -> (unsigned 16bit integer=w1206:u16)
                  }
                }
              }
            }
            n125 = Get Notifier Status(notifier=w1181) -> (notifier out=w1182:refnum<notifier>, current notification=w1180:T10)  [unwired: 1 in, 3 out]
            n126 = Bundle By Name(cluster=w1180, "Actions"=4Pi_Capture_Actions."Idle", "Frames"=w1164, "No. of Z Steps"=w1178, "Z Step Size (µm)"=w1177, "No. Amp steps"=w1165, "Amp step size"=w1176, "No. Mirror Mode"=w1172, "DM scan mode"=w1173, "Cycles"=w1170) -> (w1179:T10)
            n127 = Send Notification(notification=w1179, notifier=w1182) -> ()  [unwired: 1 in, 2 out]
            n128 = local write "No. of Cycles"(w1170) -> ()
          }
          event "Camera Settings", "Preview Exposure Time (s)", "Capture Exposure Time (s)", "No. of Cycles", "No. of Frames", "No. of Z Steps", "Z Step Size (µm)", "Base Save Path", "File Name", "Amp step size", "Mirror Mode", "No. Amp steps", "Sampling Time (s)": Value Change {
            n129 = event-data() -> ("CtlRef"=w1224:refnum<vi>)  [unwired: 1 in]
            n130 = property class="Ctl"(reference=w1224) -> ("Label.Text"=w1223:string)  [unwired: 1 in, 2 out]
            n131 = case shown="\"Mirror Mode\"" w1223 {
              tunnel: w1222 -> [_ w1229 w1237 w1243 w1249 w1254 w1260 w1270 w1274 w1301 _ w1317 w1326 w1332]
              tunnel: w1221 -> [_ _ _ _ _ _ _ _ _ _ w1309 _ _ _]
              frame Default {
              }
              frame "No. of Cycles" {
                n132 = Get Notifier Status(notifier=w1229) -> (notifier out=w1228:refnum<notifier>, current notification=w1230:T10)  [unwired: 1 in, 3 out]
                n133 = Bundle By Name(cluster=w1230, "Cycles"="No. of Cycles", "Actions"=4Pi_Capture_Actions."Idle") -> (w1231:T10)
                n134 = Send Notification(notification=w1231, notifier=w1228) -> ()  [unwired: 1 in, 2 out]
              }
              frame "No. of Frames" {
                n135 = To Double Precision Float(number="No. of Frames") -> (double precision float=w1233:dbl)
                n136 = property on="Frame" class="Slide (strict)"("Scale.Maximum"=w1233, "Scale.Minimum"=0.0 ("Scale.Range:Minimum")) -> ()  [unwired: 2 in, 2 out]
                n137 = Get Notifier Status(notifier=w1237) -> (notifier out=w1236:refnum<notifier>, current notification=w1238:T10)  [unwired: 1 in, 3 out]
                n138 = Bundle By Name(cluster=w1238, "Frames"="No. of Frames", "Actions"=4Pi_Capture_Actions."Idle") -> (w1239:T10)
                n139 = Send Notification(notification=w1239, notifier=w1236) -> ()  [unwired: 1 in, 2 out]
              }
              frame "No. of Z Steps" {
                n140 = Get Notifier Status(notifier=w1243) -> (notifier out=w1242:refnum<notifier>, current notification=w1244:T10)  [unwired: 1 in, 3 out]
                n141 = Bundle By Name(cluster=w1244, "No. of Z Steps"="No. of Z Steps", "Actions"=4Pi_Capture_Actions."Idle") -> (w1245:T10)
                n142 = Send Notification(notification=w1245, notifier=w1242) -> ()  [unwired: 1 in, 2 out]
              }
              frame "Z Step Size (µm)" {
                n143 = Get Notifier Status(notifier=w1249) -> (notifier out=w1248:refnum<notifier>, current notification=w1250:T10)  [unwired: 1 in, 3 out]
                n144 = Bundle By Name(cluster=w1250, "Z Step Size (µm)"="Z Step Size (µm)", "Actions"=4Pi_Capture_Actions."Idle") -> (w1251:T10)
                n145 = Send Notification(notification=w1251, notifier=w1248) -> ()  [unwired: 1 in, 2 out]
              }
              frame "No. Amp steps" {
                n146 = Get Notifier Status(notifier=w1254) -> (notifier out=w1256:refnum<notifier>, current notification=w1255:T10)  [unwired: 1 in, 3 out]
                n147 = Bundle By Name(cluster=w1255, "No. Amp steps"="No. Amp steps", "Actions"=4Pi_Capture_Actions."Idle") -> (w1257:T10)
                n148 = Send Notification(notification=w1257, notifier=w1256) -> ()  [unwired: 1 in, 2 out]
              }
              frame "Amp step size" {
                n149 = Get Notifier Status(notifier=w1260) -> (notifier out=w1262:refnum<notifier>, current notification=w1263:T10)  [unwired: 1 in, 3 out]
                n150 = Bundle By Name(cluster=w1263, "Amp step size"="Amp step size", "Actions"=4Pi_Capture_Actions."Idle") -> (w1261:T10)
                n151 = Send Notification(notification=w1261, notifier=w1262) -> ()  [unwired: 1 in, 2 out]
              }
              frame "Mirror Mode" {
                n152 = Array Size(array="Mirror Mode") -> (size(s)=w1268:i32)
                n153 = Get Notifier Status(notifier=w1270) -> (notifier out=w1266:refnum<notifier>, current notification=w1269:T10)  [unwired: 1 in, 3 out]
                n154 = Bundle By Name(cluster=w1269, "No. Mirror Mode"=w1268, "Actions"=4Pi_Capture_Actions."Idle") -> (w1265:T10)
                n155 = Send Notification(notification=w1265, notifier=w1266) -> ()  [unwired: 1 in, 2 out]
              }
              frame "DM scan mode" {
                n156 = local read "No. Amp steps"() -> (w1273:u16)
                n157 = local read "Mirror Mode"() -> (w1272:u16[])
                n158 = case shown="1" "DM scan mode" {
                  selector: "DM scan mode" -> [w1277 w1282]
                  tunnel: w1274 -> [w1278 w1291]
                  tunnel: w1273 -> [_ w1288]
                  tunnel: w1272 -> [_ w1289]
                  frame 0, Default {
                    n159 = Get Notifier Status(notifier=w1278) -> (notifier out=w1280:refnum<notifier>, current notification=w1279:T10)  [unwired: 1 in, 3 out]
                    n160 = Bundle By Name(cluster=w1279, "DM scan mode"=w1277, "Actions"=4Pi_Capture_Actions."Idle") -> (w1276:T10)
                    n161 = Send Notification(notification=w1276, notifier=w1280) -> ()  [unwired: 1 in, 2 out]
                  }
                  frame 1 {
                    n162 = Array Size(array=w1289) -> (size(s)=w1286:i32)
                    n163 = Get Notifier Status(notifier=w1291) -> (notifier out=w1284:refnum<notifier>, current notification=w1290:T10)  [unwired: 1 in, 3 out]
                    n164 = To Unsigned Word Integer(number=w1286) -> (unsigned 16bit integer=w1285:u16)
                    n165 = Multiply(x=w1288, y=w1285) -> (x*y=w1287:u16)
                    n166 = Bundle By Name(cluster=w1290, "Actions"=4Pi_Capture_Actions."Idle", "DM scan mode"=w1282, "Cycles"=w1287) -> (w1283:T10)
                    n167 = local write "No. of Cycles"(w1287) -> ()
                    n168 = Send Notification(notification=w1283, notifier=w1284) -> ()  [unwired: 1 in, 2 out]
                  }
                }
              }
              frame "Base Save Path", "File Name", "Save Path" {
                n169 = Path To String(path="Base Save Path") -> (string=w1296:string)
                n170 = Equal?(x="", y=w1296) -> (x = y?=w1294:bool)
                n171 = case shown="False" w1294 {
                  tunnel: [w1304 w1305] -> w1293
                  tunnel: "Base Save Path" -> [w1304 _]
                  frame False {
                  }
                  frame True {
                    w1308 = 0 items=["Desktop"=0, "Personal Documents"=5, "AppData"=26, "Local AppData"=28, "Common AppData"=35, "Program Files"=38, "Program Files Common"=43, "Common Documents"=46] ("Requested Path")
                    w1307 = 0 ("HWND")
                    n172 = dll-call lib="shell32.dll" fn="SHGetFolderPathA"("HWND"=w1307, "nFolder"=w1308, "hToken"=w1307, "dwFlags"=w1307) -> ("pszPath"=w1306:string)  [unwired: 9 in, 2 out]
                    n173 = String To Path(string=w1306) -> (path=w1305:path)
                  }
                }
                n174 = Build Path(base path=w1293, name or relative path="File Name") -> (appended path=w1297:path)
                n175 = Get Notifier Status(notifier=w1301) -> (notifier out=w1300:refnum<notifier>, current notification=w1302:T10)  [unwired: 1 in, 3 out]
                n176 = Bundle By Name(cluster=w1302, "Base Path"=w1297, "Actions"=4Pi_Capture_Actions."Idle") -> (w1303:T10)
                n177 = Send Notification(notification=w1303, notifier=w1300) -> ()  [unwired: 1 in, 2 out]
              }
              frame "Camera Settings" {
                n178 = Select(t=Common_Device_Actions."Open Front Panel" ("Common Actions"), s="Camera Settings", f=Common_Device_Actions."Close Front Panel" ("Common Actions")) -> (s? t:f=w1313:T34)
                n179 = call "Common Device Queue Messenger.vi"("Common Action"=w1313, "Notifier Name"=w1309) -> ()  [unwired: 13 in, 1 out]
              }
              frame "Preview Exposure Time (s)" {
                # "Add in a preview stop\nand restart here"
                n180 = Get Notifier Status(notifier=w1317) -> (notifier out=w1320:refnum<notifier>, current notification=w1319:T10)  [unwired: 1 in, 3 out]
                n181 = Bundle By Name(cluster=w1319, "Preview Exposure (s)"="Preview Exposure Time (s)", "Running?"=FALSE ("Abort"), "Actions"=4Pi_Capture_Actions."Idle") -> (w1318:T10)
                n182 = Send Notification(notification=w1318, notifier=w1320) -> ()  [unwired: 1 in, 2 out]
              }
              frame "Capture Exposure Time (s)" {
                n183 = Get Notifier Status(notifier=w1326) -> (notifier out=w1325:refnum<notifier>, current notification=w1324:T10)  [unwired: 1 in, 3 out]
                n184 = Bundle By Name(cluster=w1324, "Capture Exposure (s)"="Capture Exposure Time (s)", "Actions"=4Pi_Capture_Actions."Idle") -> (w1323:T10)
                n185 = Send Notification(notification=w1323, notifier=w1325) -> ()  [unwired: 1 in, 2 out]
              }
              frame "Sampling Time (s)" {
                n186 = Get Notifier Status(notifier=w1332) -> (notifier out=w1331:refnum<notifier>, current notification=w1330:T10)  [unwired: 1 in, 3 out]
                n187 = Bundle By Name(cluster=w1330, "Sampling Time (s)"="Sampling Time (s)", "Actions"=4Pi_Capture_Actions."Idle") -> (w1329:T10)
                n188 = Send Notification(notification=w1329, notifier=w1331) -> ()  [unwired: 1 in, 2 out]
              }
            }
          }
          event "Live Preview", "Capture": Value Change {
            n189 = event-data() -> ("CtlRef"=w1336:refnum<vi>, "NewVal"=w1339:bool)  [unwired: 1 in]
            n190 = property class="Bool (strict)"(reference=w1336) -> ("Label.Text"=w1335:string)  [unwired: 1 in, 2 out]
            n191 = case shown="\"Capture\"" w1335 {
              tunnel: [4Pi_Capture_Actions."Capture" ("y") 4Pi_Capture_Actions."Live Preview" ("y")] -> w1334
              frame "Capture" {
              }
              frame "Live Preview", Default {
              }
            }
            n192 = Select(t=w1334, s=w1339, f=4Pi_Capture_Actions."Abort" ("y")) -> (s? t:f=w1338:T11)
            n193 = Get Notifier Status(notifier=w1341) -> (notifier out=w1342:refnum<notifier>, current notification=w1340:T10)  [unwired: 1 in, 3 out]
            n194 = Bundle By Name(cluster=w1340, "Actions"=w1338, "Running?"=w1339) -> (w1337:T10)
            n195 = Send Notification(notification=w1337, notifier=w1342) -> ()  [unwired: 1 in, 2 out]
          }
          event "Quadrants On/Off": Value Change {
            n196 = event-data() -> ("NewVal"=w1361:bool)  [unwired: 1 in]
            n197 = Obtain Notifier(name (unnamed)="Display Module IMAQ Refs", notification data type=T6[] [], create if not found? (T)=FALSE) -> (notifier out=w1354:refnum<notifier>, error out=w1353:errorcluster)  [unwired: 1 in, 1 out]
            n198 = Get Notifier Status(notifier=w1354, error in (no error)=w1353) -> (notifier out=w1352:refnum<notifier>, current notification=w1350:T6[], error out=w1351:errorcluster)  [unwired: 2 out]
            n199 = case shown="True" w1361 {
              tunnel: w1352 -> [w1387 w1402]
              tunnel: w1351 -> [w1386 w1401]
              tunnel: [w1383 w1397] -> w1357
              tunnel: [w1387 w1402] -> w1358
              tunnel: [w1386 w1401] -> w1356
              tunnel: w1355 -> [w1378 w1400]
              tunnel: w1350 -> [w1385 w1399]
              tunnel: w1349 -> [w1379 w1396]
              tunnel: w1348 -> [_ w1395]
              tunnel: [w1366 w1395] -> w1347
              frame False {
                w1377 = 4 ("dimension size")
                n200 = control-ref of="This VI"() -> (w1367:refnum<vi>)
                n201 = Equal?(x=w1385, y=w1379) -> (x = y?=w1382:bool[])
                n202 = property class="VI"(reference=w1367) -> (error out=w1375:errorcluster, "Path"=w1368:path)  [unwired: 1 in, 1 out]
                n203 = for {
                  tunnel: w1382 -> [w1394] mode=indexing
                  tunnel: [w1393] -> w1380
                  i -> [w1393]
                  stop <- w1394 stop-if-true
                }
                n204 = Or Array Elements(Boolean array=w1382) -> (logical OR=w1381:bool)
                n205 = Strip Path(path=w1368) -> (stripped path=w1374:path)  [unwired: 1 out]
                n206 = case shown="True" w1381 {
                  tunnel: w1380 -> [_ w1391]
                  tunnel: w1385 -> [w1388 w1390]
                  tunnel: [w1388 w1389] -> w1384
                  frame False {
                  }
                  frame True {
                    n207 = Delete From Array(array=w1390, length=1, index=w1391) -> (array with subset deleted=w1389:T6[])  [unwired: 1 out]
                  }
                }
                n208 = Build Path(base path=w1374, name or relative path="Quadrant Coordinates Array.txt") -> (appended path=w1372:path)
                n209 = Read from Text File(file (use dialog)=w1372, error in=w1375) -> (text=w1373:string, error out=w1376:errorcluster)  [unwired: 2 in, 2 out]
                n210 = Initialize Array(0 ("element"), w1377, w1377) -> (w1371:i32[][])
                n211 = Build Array (concatenate)(w1384, w1378) -> (w1383:T6[])
                n212 = Unflatten From JSON(JSON string=w1373, type and defaults=w1371, error in (no error)=w1376) -> (value=w1366:i32[][])  [unwired: 4 in, 1 out]
              }
              frame True {
                n213 = for {
                  tunnel: w1400 -> [w1405] mode=indexing
                  shift-right: [w1403] -> w1398
                  shift-left: w1399 -> [w1404]
                  n214 = Equal?(x=w1404, y=w1405) -> (x = y?=w1408:bool[])
                  n215 = for {
                    tunnel: w1408 -> [w1415] mode=indexing
                    tunnel: [w1414] -> w1406
                    i -> [w1414]
                    stop <- w1415 stop-if-true
                  }
                  n216 = Or Array Elements(Boolean array=w1408) -> (logical OR=w1407:bool)
                  n217 = case shown="True" w1407 {
                    tunnel: w1406 -> [_ w1412]
                    tunnel: w1404 -> [w1409 w1411]
                    tunnel: [w1409 w1410] -> w1403
                    frame False {
                    }
                    frame True {
                      n218 = Delete From Array(array=w1411, length=1, index=w1412) -> (array with subset deleted=w1410:T6[])  [unwired: 1 out]
                    }
                  }
                }
                n219 = Build Array (concatenate)(w1398, w1396) -> (w1397:T6[])
              }
            }
            n220 = Send Notification(notification=w1357, notifier=w1358, error in (no error)=w1356) -> (notifier out=w1360:refnum<notifier>, error out=w1359:errorcluster)
            n221 = Release Notifier(notifier=w1360, error in (no error)=w1359) -> ()  [unwired: 1 in, 3 out]
          }
          event "Auto Update Subfolder": Value Change {
            n222 = event-data() -> ("NewVal"=w1420:bool)  [unwired: 1 in]
            n223 = Select(t=T8."Enabled" ("Disabled"), s=w1420, f=T8."Disabled and Grayed Out") -> (s? t:f=w1417:T8)
            n224 = property on="Subfolder Name" class="Str"("DisabledEnum"=w1417) -> ()  [unwired: 2 in, 2 out]
          }
          event "Line Scan Active": Value Change {
            n225 = event-data() -> ("NewVal"=w1422:bool)  [unwired: 1 in]
            n226 = Select(t="Frame Rate (Hz)", s=w1422, f="Exposure Time (s)") -> (s? t:f=w1443:string)
            n227 = Select(t=4.0, s=w1422, f=0.1) -> (s? t:f=w1436:dbl)
            n228 = Select(t=-1.0 ("f"), s=w1422, f=0.0) -> (s? t:f=w1427:dbl)
            n229 = Select(t=AO_SCTR_Actions."Update and Run" ("Actions"), s=w1422, f=AO_SCTR_Actions."Stop at Offset" ("Actions")) -> (s? t:f=w1428:T30)
            n230 = property on="Capture Exposure Time (s)" class="DigNum (strict)"("Caption.Text"=w1443, "Value"=w1436) -> ()  [unwired: 2 in, 2 out]
            n231 = property on="Preview Exposure Time (s)" class="DigNum (strict)"("Caption.Text"=w1443, "Value"=w1436) -> ()  [unwired: 2 in, 2 out]
            n232 = call "AO SCTR Messenger.vi"("Notifier Name"=w1424, "Actions"=w1428, "Offset (V)"=w1427) -> ()  [unwired: 12 in, 1 out]
            n233 = case shown="False" w1422 {
              frame False {
                w1447 = T8."Enabled" ("Disabled")
                n234 = property on="Preview Exposure Time (s)" class="DigNum (strict)"("DisabledEnum"=w1447) -> ()  [unwired: 2 in, 2 out]
                n235 = property on="Capture Exposure Time (s)" class="DigNum (strict)"("DisabledEnum"=w1447) -> ()  [unwired: 2 in, 2 out]
              }
              frame True {
              }
            }
            n236 = Get Notifier Status(notifier=w1440) -> (notifier out=w1439:refnum<notifier>, current notification=w1438:T10)  [unwired: 1 in, 3 out]
            n237 = Bundle By Name(cluster=w1438, "Line Scan?"=w1422, "Actions"=4Pi_Capture_Actions."Idle", "Preview Exposure (s)"=w1436, "Capture Exposure (s)"=w1436) -> (w1435:T10)
            n238 = Select(t=Orca_Flash_Actions."PROGRESSIVE MODE" ("Camera Actions"), s=w1422, f=Orca_Flash_Actions."AREA MODE" ("Camera Actions")) -> (s? t:f=w1431:T21)
            n239 = call "Orca Flash Messanger.vi"("Notifier Name"=w1434, "Camera Actions"=w1431) -> ()  [unwired: 9 in, 5 out]
            n240 = Send Notification(notification=w1435, notifier=w1439) -> ()  [unwired: 1 in, 2 out]
          }
          event Value Change {
            n241 = event-data() -> ("NewVal"=w1457:T3)  [unwired: 1 in]
            n242 = Get Notifier Status(notifier=w1466) -> (notifier out=w1465:refnum<notifier>, current notification=w1464:T10)  [unwired: 1 in, 3 out]
            n243 = Bundle By Name(cluster=w1464, "Actions"=4Pi_Capture_Actions."Idle", "Line Scan Mode"=w1457) -> (w1463:T10)
            n244 = Send Notification(notification=w1463, notifier=w1465) -> ()  [unwired: 1 in, 2 out]
            n245 = Equal?(x=w1457, y=4Pi_Capture_Switch_Line_Scan_Modes."Use Presets") -> (x = y?=w1449:bool)
            n246 = Not Equal?(x=w1457, y=4Pi_Capture_Switch_Line_Scan_Modes."Automatic") -> (x != y?=w1451:bool)
            n247 = Select(t=T8."Enabled" ("Disabled"), s=w1449, f=T8."Disabled and Grayed Out" ("Disabled")) -> (s? t:f=w1459:T8)
            n248 = property on="Line Scanning Presets" class="Ring (strict)"("DisabledEnum"=w1459) -> ()  [unwired: 2 in, 2 out]
            n249 = case shown="True" w1449 {
              frame False {
              }
              frame True {
                n250 = property on="Line Scanning Presets" class="Ring (strict)"() -> ("Value"=w1469:u16)  [unwired: 2 in, 2 out]
                n251 = property on="Line Scanning Presets" class="Ring (strict)"("Val(Sgnl)"=w1469) -> ()  [unwired: 2 in, 2 out]
              }
            }
            n252 = Select(t=T8."Disabled and Grayed Out" ("Disabled"), s=w1451, f=T8."Enabled" ("Disabled")) -> (s? t:f=w1450:T8)
            n253 = Select(t=T8."Enabled" ("Disabled"), s=w1451, f=T8."Disabled and Grayed Out" ("Disabled")) -> (s? t:f=w1454:T8)
            n254 = property on="Preview Exposure Time (s)" class="DigNum (strict)"("DisabledEnum"=w1450) -> ()  [unwired: 2 in, 2 out]
            n255 = property on="Capture Exposure Time (s)" class="DigNum (strict)"("DisabledEnum"=w1450) -> ()  [unwired: 2 in, 2 out]
            n256 = property on="Save As Preset" class="Bool"("DisabledEnum"=w1454) -> ()  [unwired: 2 in, 2 out]
            n257 = property on="Line Scan Settings" class="Clust (strict)"("DisabledEnum"=w1454) -> ()  [unwired: 2 in, 2 out]
          }
          event "Line Scanning Presets": Value Change {
            n258 = event-data() -> ("CtlRef"=w1479:refnum<vi>)  [unwired: 1 in]
            n259 = control-ref of="This VI"() -> (w1483:refnum<vi>)
            n260 = property class="Ring (strict)"(reference=w1479) -> ("RingText.Text"=w1477:string)  [unwired: 1 in, 2 out]
            n261 = property class="VI"(reference=w1483) -> ("Path"=w1482:path)  [unwired: 1 in, 2 out]
            n262 = Strip Path(path=w1482) -> (stripped path=w1481:path)  [unwired: 1 out]
            n263 = Concatenate Strings(w1477, ".json" ("string")) -> (w1475:string)
            n264 = Build Path(base path=w1481, name or relative path="4Pi Capture Manager Line Scan Presets") -> (appended path=w1478:path)
            n265 = Build Path(base path=w1478, name or relative path=w1475) -> (appended path=w1474:path)
            n266 = Read from Text File(file (use dialog)=w1474) -> (text=w1473:string, error out=w1471:errorcluster)  [unwired: 3 in, 2 out]
            n267 = Unflatten From JSON(JSON string=w1473, type and defaults=T4 {"Interline Interval"=0.0, "Offset (V)"=0.0, "Amplitude (V)"=0.0, "Samples Per Channel"=0.0, "Delay (ms)"=0.0} ("Line Scan Settings"), error in (no error)=w1471) -> (value=w1470:T4)  [unwired: 4 in, 1 out]
            n268 = property on="Line Scan Settings" class="Clust (strict)"("Val(Sgnl)"=w1470) -> ()  [unwired: 2 in, 2 out]
          }
          event Value Change {
            # "If you try and set the ILI while the camera is in area mode it gives an error"
            n269 = event-data() -> ("NewVal"=w1497:T4)  [unwired: 1 in]
            n270 = Get Notifier Status(notifier=w1502) -> (current notification=w1501:T10)  [unwired: 1 in, 4 out]
            n271 = Unbundle By Name(w1497) -> ("Offset (V)"=w1491:dbl, "Amplitude (V)"=w1495:dbl, "Samples Per Channel"=w1494:dbl, "Delay (ms)"=w1493:dbl, "Interline Interval"=w1487:dbl)
            n272 = Unbundle By Name(w1501) -> ("Line Scan?"=w1486:bool)
            n273 = To Long Integer(number=w1494) -> (32bit integer=w1492:i32)
            n274 = Select(t=w1491, s=w1486, f=0.0) -> (s? t:f=w1489:dbl)
            n275 = Select(t=AO_SCTR_Actions."Update and Run" ("Actions"), s=w1486, f=AO_SCTR_Actions."Stop at Offset" ("Actions")) -> (s? t:f=w1498:T30)
            n276 = call "AO SCTR Messenger.vi"("Notifier Name"=w1496, "Actions"=w1498, "Offset (V)"=w1489, "Amplitude (V)"=w1495, "Samples Per Channel"=w1492, "Start Delay (ms)"=w1493) -> ()  [unwired: 9 in, 1 out]
            n277 = case shown="True" w1486 {
              tunnel: w1488 -> [_ w1507]
              tunnel: w1487 -> [_ w1506]
              frame False {
              }
              frame True {
                n278 = Bundle By Name(cluster=T17 {"Value"=0.0, "Parameter"=4226016} ("sCMOS Parameter"), "Value"=w1506) -> (w1510:T17)
                n279 = call "Orca Flash Messanger.vi"("Notifier Name"=w1507, "Camera Actions"=Orca_Flash_Actions."SETPARAM", "sCMOS Parameter"=w1510) -> ("sCMOS Parameter"=w1511:T17)  [unwired: 8 in, 4 out]
                n280 = Unbundle By Name(w1511) -> ("Value"=w1505:dbl)
                n281 = property on="Interline Interval" class="DigNum (strict)"("Value"=w1505) -> ()  [unwired: 2 in, 2 out]
              }
            }
          }
          event "Save As Preset": Value Change {
            n282 = event-data() -> ()  [unwired: 1 in, 6 out]
            n283 = control-ref of="This VI"() -> (w1524:refnum<vi>)
            n284 = property class="VI"(reference=w1524) -> ("Path"=w1523:path)  [unwired: 1 in, 2 out]
            n285 = Strip Path(path=w1523) -> (stripped path=w1522:path)  [unwired: 1 out]
            n286 = Build Path(base path=w1522, name or relative path="4Pi Capture Manager Line Scan Presets") -> (appended path=w1513:path)
            n287 = call "File Dialog"("start path"=w1513, "prompt"="Save Preset File", "pattern (all files)"="*.json", "pattern label"="JSON") -> ("selected path"=w1518:path, "error out"=w1519:errorcluster)  [unwired: 8 in, 2 out]
            n288 = case shown="Error" w1519 {
              selector: w1519 -> [_ w1542]
              tunnel: w1518 -> [w1541 _]
              tunnel: [w1537 w1542] -> w1512
              frame No Error {
                n289 = local read "Line Scan Settings"() -> (w1540:T4)
                n290 = Flatten To JSON(anything=w1540) -> (JSON string=w1539:string, 11:w1538:errorcluster)  [unwired: 2 in]
                n291 = Write to Text File(file (use dialog)=w1541, text=w1539, error in=w1538) -> (error out=w1537:errorcluster)  [unwired: 1 in, 2 out]
              }
              frame Error {
              }
            }
            n292 = List Folder(path=w1513, pattern="*.json", error in=w1512) -> (filenames=w1516:string[], error out=w1515:errorcluster)  [unwired: 1 in, 2 out]
            n293 = case shown="No Error" w1515 {
              tunnel: w1516 -> [w1531 _]
              tunnel: w1513 -> [w1530 _]
              tunnel: [w1529 string[] []] -> w1514
              frame No Error {
                n294 = for {
                  tunnel: w1531 -> [w1534] mode=indexing
                  tunnel: w1530 -> [w1535]
                  tunnel: [w1532] -> w1529 mode=indexing
                  n295 = Build Path(base path=w1535, name or relative path=w1534) -> (appended path=w1533:path)
                  n296 = call <vilib>:"Get File Extension.vi"("file"=w1533) -> ("filename without extension"=w1532:string)  [unwired: 6 in, 4 out]
                }
              }
              frame Error {
              }
            }
            n297 = property on="Line Scanning Presets" class="Ring (strict)"("Strings []"=w1514) -> ()  [unwired: 2 in, 2 out]
          }
          event "Quit": Value Change {
            n298 = event-data() -> ("NewVal"=w1557:bool)  [unwired: 1 in]
            n299 = Get Notifier Status(notifier=w1556) -> (notifier out=w1555:refnum<notifier>, current notification=w1554:T10)  [unwired: 1 in, 3 out]
            n300 = Bundle By Name(cluster=w1554, "Running?"=FALSE ("Abort"), "Actions"=4Pi_Capture_Actions."Quit") -> (w1548:T10)
            n301 = Send Notification(notification=w1548, notifier=w1555) -> (notifier out=w1552:refnum<notifier>)  [unwired: 1 in, 1 out]
            n302 = Wait on Notification(notifier=w1552, ignore previous (F)=TRUE, timeout in ms (-1)=500) -> (notifier out=w1549:refnum<notifier>)  [unwired: 1 in, 3 out]
            n303 = Send Notification(notification=w1548, notifier=w1549) -> (notifier out=w1546:refnum<notifier>)  [unwired: 1 in, 1 out]
            n304 = Release Notifier(notifier=w1546, force destroy? (F)=TRUE) -> ()  [unwired: 1 in, 3 out]
            n305 = for {
              tunnel: w1544 -> [w1558] mode=indexing
              n306 = call "IMAQ Dispose"("Image"=w1558) -> ()  [unwired: 5 in, 1 out]
            }
          }
        }
      }
      n307 = while {
        tunnel: w211 -> [w254]
        tunnel: w180 -> [w248]
        tunnel: w210 -> [w246]
        tunnel: w209 -> [w245]
        tunnel: w208 -> [w244]
        tunnel: [FALSE] -> w207
        tunnel: w201 -> [w242]
        tunnel: w174 -> [w237]
        tunnel: w173 -> [w236]
        tunnel: w165 -> [w235]
        tunnel: [w235] -> w164
        tunnel: w152 -> [w232]
        stop <- w250 stop-if-true
        w233 = u16 0 ("Current Mode")
        w240 = u16 0 ("Current Step")
        n308 = Wait on Notification(notifier=w254, ignore previous (F)=TRUE) -> (notifier out=w249:refnum<notifier>, notification=w252:T10)  [unwired: 2 in, 2 out]
        n309 = Unbundle By Name(w252) -> ("Actions"=w247:T11)
        n310 = Bundle By Name(cluster=T22 {"Current Step"=0, "Current Cycle"=0, "Current Laser"=0, "# of Lasers"=0, "# of Cycles"=0, "# of Steps"=0, "Switch Laser At"=enum."All Cycles", "Current Mirror Mode"=0, "# of Mirror Mode"=0, "Current Amp step"=0, "# of Amp steps"=0} ("Cluster"), "Current Step"=w240, "Current Cycle"=w240, "Current Laser"=w240, "# of Lasers"=u16 1, "Switch Laser At"="Switch Laser At", "Current Mirror Mode"=w233, "Current Amp step"=w233) -> (w239:T22)
        n311 = Equal?(x=w247, y=4Pi_Capture_Actions."Quit") -> (x = y?=w250:bool)
        n312 = while {
          shift-right: [w270] -> _
          shift-left: w247 -> [w271]
          tunnel: w249 -> [w262]
          tunnel: w248 -> [w267]
          tunnel: w247 -> [w266]
          tunnel: w246 -> [w265]
          tunnel: w245 -> [w264]
          tunnel: w244 -> [w263]
          tunnel: w242 -> [w261]
          shift-right: [w259] -> _
          shift-left: w239 -> [w260]
          tunnel: w237 -> [w258]
          tunnel: w236 -> [w257]
          tunnel: w235 -> [w256]
          tunnel: w232 -> [w255]
          stop <- w268 stop-if-true
          n313 = case shown="\"Start Acquisition\"" w271 {
            selector: w271 -> [_ _ _ w370 w398 _ _ _ _ _ _ _ _ _ _ _ _ _ _]
            tunnel: [4Pi_Capture_Actions."Quit" ("y") 4Pi_Capture_Actions."Open Shutters" ("y") 4Pi_Capture_Actions."Close Shutters" ("y") w361 w392 4Pi_Capture_Actions."Start Acquisition" ("y") w460 4Pi_Capture_Actions."Write Metadata" ("y") w567 w624 w658 w703 w797 w829 w857 w934 w987 w1106 4Pi_Capture_Actions."Quit" ("y")] -> w270
            tunnel: [w273 w285 w323 w372 w396 w419 w462 w539 w599 w633 w667 w733 w823 w828 w872 w953 w1004 w1128 TRUE] -> w268
            tunnel: FALSE -> [w273 w285 w323 w372 w396 w419 w462 w539 w599 w633 w667 w733 w823 w828 w872 w953 w1004 w1128 _]
            tunnel: w267 -> [_ w278 w317 _ _ w404 w461 _ _ _ w657 w725 _ _ _ _ _ _ _]
            tunnel: w266 -> [_ _ w316 _ _ w412 w458 w536 w591 _ _ _ _ _ _ _ _ _ _]
            tunnel: w265 -> [_ _ _ _ w395 _ _ _ _ _ _ _ _ _ _ _ _ _ _]
            tunnel: w264 -> [_ _ _ w371 _ _ _ _ _ _ _ _ _ _ _ _ _ _ _]
            tunnel: w263 -> [_ _ _ w366 _ _ _ _ _ _ _ _ _ _ _ _ _ _ _]
            tunnel: w262 -> [_ _ w314 _ _ w417 w459 w538 w592 _ w659 w726 w803 _ w871 w952 w1003 _ _]
            tunnel: w261 -> [_ _ w311 _ _ _ w457 _ _ _ _ _ _ _ w869 w945 _ _ _]
            tunnel: w260 -> [w272 w284 w295 w359 w390 w407 w456 w537 w564 w632 w652 w701 w801 w836 w862 w939 w994 w1127 w1150]
            tunnel: [w272 w284 w295 w359 w390 w407 w455 w537 w564 w632 w652 w700 w822 w835 w862 w939 w994 w1127 w1150] -> w259
            tunnel: w258 -> [_ _ _ _ _ w400 _ _ _ _ _ _ _ _ _ _ _ _ _]
            tunnel: w257 -> [_ _ _ _ _ w399 _ _ _ _ _ _ _ _ _ _ _ _ _]
            tunnel: w256 -> [_ w283 w290 _ _ _ w454 _ _ _ w647 w718 _ _ _ w943 _ _ _]
            tunnel: w255 -> [_ _ _ _ _ _ w453 _ _ _ _ _ _ _ _ _ _ _ _]
            frame "Idle", Default {
            }
            frame "Live Preview", "Capture" {
              w275 = FALSE ("Camera Running?")
              n314 = call "Orca Flash Messanger.vi"("Notifier Name"=w278, "Camera Actions"=Orca_Flash_Actions."STATUS") -> ("Image Ref"=w277:T6)  [unwired: 9 in, 4 out]
              n315 = Get Notifier Status(notifier=w283) -> (notifier out=w281:refnum<notifier>, current notification=w282:T7)  [unwired: 1 in, 3 out]
              n316 = Bundle By Name(cluster=w282, "Image Ref"=w277, "Cycle Number"=u16 0, "Camera Running?"=w275, "Capture?"=w275) -> (w280:T7)
              n317 = Send Notification(notification=w280, notifier=w281) -> ()  [unwired: 1 in, 2 out]
            }
            frame "Abort" {
              w294 = FALSE ("Capture?")
              w310 = u16 1 ("Current Cycle")
              w318 = FALSE ("Live Preview")
              n318 = call "Orca Flash Messanger.vi"("Notifier Name"=w317, "Camera Actions"=Orca_Flash_Actions."IDLE") -> ()  [unwired: 9 in, 5 out]
              n319 = local write "Live Preview"(w318) -> ()
              n320 = local write "Capture"(w318) -> ()
              n321 = Equal?(x=4Pi_Capture_Actions."Capture", y=w316) -> (x = y?=w296:bool)
              n322 = Get Notifier Status(notifier=w314) -> (notifier out=w321:refnum<notifier>, current notification=w320:T10)  [unwired: 1 in, 3 out]
              n323 = Bundle By Name(cluster=w320, "Running?"=FALSE) -> (w313:T10)
              n324 = local write "Current Cycle"(w310) -> ()
              n325 = local write "Current Step"(w310) -> ()
              n326 = Get Notifier Status(notifier=w290) -> (notifier out=w293:refnum<notifier>, current notification=w292:T7)  [unwired: 1 in, 3 out]
              n327 = Bundle By Name(cluster=w292, "Camera Running?"=w294, "Capture?"=w294) -> (w291:T7)
              n328 = Send Notification(notification=w313, notifier=w321) -> ()  [unwired: 1 in, 2 out]
              n329 = Unbundle By Name(w313) -> ("Init Mirror Modes"=w287:T12, "Metadata File Ref"=w288:refnum<file>[], "Init Z Position (µm)"=w312:dbl)
              n330 = Obtain Notifier(name (unnamed)="WFDC External Sync", notification data type=T24 {"Cycle Sync"=enum."Pause Requested", "Z Offset"=0.0, "WFDC Status"=enum."Idle"} ("WFDC External Sync"), create if not found? (T)=FALSE) -> (notifier out=w306:refnum<notifier>, error out=w300:errorcluster)  [unwired: 1 in, 1 out]
              n331 = Send Notification(notification=w291, notifier=w293) -> ()  [unwired: 1 in, 2 out]
              n332 = Get Notifier Status(notifier=w306, error in (no error)=w300) -> (notifier out=w298:refnum<notifier>, current notification=w297:T24, error out=w301:errorcluster)  [unwired: 2 out]
              n333 = Unbundle By Name(w297) -> ("WFDC Status"=w305:T23)
              n334 = Unbundle By Name(w301) -> ("status"=w302:bool)
              n335 = Not A Number/Path/Refnum?(number/path/refnum=w288) -> (NaN/Path/Refnum?=w289:bool[])
              n336 = for {
                tunnel: w289 -> [w326] mode=indexing
                tunnel: w288 -> [w325] mode=indexing
                n337 = case shown="False" w326 {
                  tunnel: w325 -> [w327 _]
                  frame False {
                    n338 = Close File(refnum=w327) -> ()  [unwired: 1 in, 2 out]
                  }
                  frame True {
                  }
                }
              }
              n339 = Not Equal?(x=WFDC_Status."DC Active", y=w305) -> (x != y?=w303:bool)
              n340 = Or(x=w303, y=w302) -> (x .or. y?=w299:bool)
              n341 = case shown="True" w296 {
                tunnel: w312 -> [_ w337]
                tunnel: w311 -> [_ w336]
                tunnel: w299 -> [_ w335]
                tunnel: w298 -> [_ w334]
                tunnel: w297 -> [_ w333]
                tunnel: w287 -> [_ w328]
                frame False {
                }
                frame True {
                  w329 = 4Pi_Dual_DM_-_Standard_Action."Read" ("Action")
                  n342 = case shown="True" w335 {
                    tunnel: w337 -> [_ w358]
                    tunnel: w336 -> [_ w357]
                    tunnel: w334 -> [w351 _]
                    tunnel: w333 -> [w350 _]
                    frame False {
                      n343 = Bundle By Name(cluster=w350, "Z Offset"=0.0) -> (w352:T24)
                      n344 = Send Notification(notification=w352, notifier=w351) -> (notifier out=w347:refnum<notifier>)  [unwired: 1 in, 1 out]
                      n345 = Release Notifier(notifier=w347, force destroy? (F)=FALSE) -> ()  [unwired: 1 in, 3 out]
                    }
                    frame True {
                      n346 = Build Array(w358) -> (w353:dbl[])
                      n347 = call "Stages Messenger.vi"("Stage Notifier Name"=w357, "Actions"=Stage_Actions."MOVE", "Setpoint"=w353, "Axis"=bool[] [TRUE], "Exit While Busy?"=FALSE) -> ()  [unwired: 6 in, 5 out]
                    }
                  }
                  n348 = call "4Pi Dual DM - Mirror Mode DUAL AE.vi"("Action"=w329) -> ("Mirror Modes Out"=w331:T35)  [unwired: 14 in]
                  n349 = call "4Pi Dual DM - Active Mirror AE.vi"("Action"=w329) -> ("Active Mirror"=w330:i32)  [unwired: 14 in]
                  n350 = Replace Array Subset(array=w331, new element=w328, index (col)=w330) -> (w332:T35)  [unwired: 1 in]
                  n351 = flat-sequence {
                    tunnel: w332 -> [w338]
                    frame #0 {
                      n352 = call "4Pi Dual DM - Mirror Mode DUAL AE.vi"("Action"=4Pi_Dual_DM_-_Standard_Action."Write", "Mirror Modes In"=w338) -> ()  [unwired: 13 in, 1 out]
                    }
                    frame #1 {
                      w344 = "Mirror Control Que" ("name (unnamed)")
                      n353 = Obtain Queue(max queue size (-1, unlimited)=10, name (unnamed)=w344, element data type=w344, create if not found? (T)=FALSE) -> (queue out=w340:refnum<queue>, error out=w341:errorcluster)  [unwired: 1 in, 1 out]
                      n354 = case shown="No Error" w341 {
                        tunnel: w340 -> [w345 _]
                        frame No Error {
                          n355 = Enqueue Element(queue=w345, element="Mirror Modes" ("name (unnamed)")) -> ()  [unwired: 2 in, 3 out]
                        }
                        frame Error {
                        }
                      }
                    }
                  }
                }
              }
            }
            frame "Open Shutters", "Close Shutters" {
              n356 = Equal?(x=w370, y=4Pi_Capture_Actions."Open Shutters") -> (x = y?=w364:bool)
              n357 = Select(t=Shutter_Actions."Open" ("Action"), s=w364, f=Shutter_Actions."Close") -> (s? t:f=w365:T28)
              n358 = case shown="False" "Auto Shutter" {
                tunnel: w371 -> [_ w379]
                tunnel: w366 -> [_ w374]
                tunnel: w365 -> [_ w373]
                frame False {
                }
                frame True {
                  n359 = flat-sequence {
                    tunnel: w373 -> [w382]
                    tunnel: w379 -> [w383]
                    tunnel: [w383] -> w376
                    tunnel: [w382] -> w375
                    tunnel: w374 -> [w381]
                    tunnel: w373 -> [w380]
                    tunnel: [w386] -> w378
                    tunnel: [w385] -> w377
                    tunnel: w376 -> [w386]
                    tunnel: w375 -> [w385]
                    tunnel: w378 -> [w388]
                    tunnel: w377 -> [w387]
                    frame #0 {
                      n360 = call "Shutter Messenger.vi"("Notifier Name"=w381, "Action"=w380) -> ()  [unwired: 12 in, 2 out]
                    }
                    frame #1 {
                      n361 = Wait (ms)(milliseconds to wait=u32 100) -> ()  [unwired: 1 out]
                    }
                    frame #2 {
                      n362 = call "Shutter Messenger.vi"("Notifier Name"=w388, "Action"=w387) -> ()  [unwired: 12 in, 2 out]
                    }
                  }
                }
              }
              n363 = Select(t=4Pi_Capture_Actions."Laser On" ("y"), s=w364, f=4Pi_Capture_Actions."Laser Off") -> (s? t:f=w361:T11)
            }
            frame "Laser On", "Laser Off" {
              n364 = Equal?(x=w398, y=4Pi_Capture_Actions."Laser On") -> (x = y?=w389:bool)
              n365 = call "AOTF Messenger.vi"("AOTF Notifier Name"=w395, "AOTF Action"=AOTF_Actions."Blank", "Beam Blank"=w389) -> ()  [unwired: 7 in, 6 out]
              n366 = Select(t=4Pi_Capture_Actions."Set Exposure Time" ("y"), s=w389, f=4Pi_Capture_Actions."Quit" ("y")) -> (s? t:f=w392:T11)
            }
            frame "Set Exposure Time" {
              # "Frame Rate (Hz)"
              n367 = Get Notifier Status(notifier=w417) -> (current notification=w413:T10)  [unwired: 1 in, 4 out]
              n368 = Unbundle By Name(w413) -> ("Line Scan?"=w402:bool, "Line Scan Mode"=w401:T3, "Capture Exposure (s)"=w408:dbl, "Preview Exposure (s)"=w409:dbl)
              n369 = Equal?(x=w412, y=4Pi_Capture_Actions."Capture") -> (x = y?=w410:bool)
              n370 = Select(t=w408, s=w410, f=w409) -> (s? t:f=w406:dbl)
              n371 = case shown="True" w402 {
                tunnel: w406 -> [w421 w429]
                tunnel: [w421 w426] -> w405
                tunnel: w404 -> [w420 w428]
                tunnel: [w420 w425] -> w403
                tunnel: w401 -> [_ w424]
                tunnel: w400 -> [_ w423]
                tunnel: w399 -> [_ w422]
                frame False {
                  # "Exposure Time (s)"
                }
                frame True {
                  n372 = To Double Precision Float(number="Number of Lines") -> (double precision float=w427:dbl)
                  n373 = case shown="Default" w424 {
                    tunnel: w429 -> [_ w452]
                    tunnel: w428 -> [w435 w451]
                    tunnel: w427 -> [w433 w450]
                    tunnel: [w431 w449] -> w426
                    tunnel: [w434 w448] -> w425
                    tunnel: w423 -> [_ w441]
                    tunnel: w422 -> [_ w440]
                    frame Default {
                      n374 = call "Orca Flash Messanger.vi"("Notifier Name"=w435, "Camera Actions"=Orca_Flash_Actions."GETPARAM", "sCMOS Parameter"=T17 {"Value"=0.0, "Parameter"=4226016}) -> ("Notifier Name Dup"=w434:string, "sCMOS Parameter"=w438:T17)  [unwired: 8 in, 3 out]
                      n375 = Unbundle By Name(w438) -> ("Value"=w432:dbl)
                      n376 = Multiply(x=w432, y=w433) -> (x*y=w431:dbl)
                    }
                    frame "Automatic" {
                      n377 = call "4Pi Capture Set Interline Interval.vi"("Camera Notifier Name"=w451, "Frame Rate (Hz)"=w452) -> ("Camera Notifier Name (Dup)"=w448:string, "Interline Interval (s)"=w447:dbl)  [unwired: 12 in]
                      n378 = Multiply(x=w447, y=w450) -> (x*y=w449:dbl)
                      n379 = call "4Pi Capture Set Auto Waveform.vi"("Interline Interval"=w447, "Waveform Parameters"=w440) -> ("Offset (V)"=w445:dbl, "Amplitude (V)"=w444:dbl, "Samples per Channel"=w443:i32, "Delay (ms)"=w442:dbl, "Line Scan Settings"=w439:T4)  [unwired: 9 in]
                      n380 = local write "Line Scan Settings"(w439) -> ()
                      n381 = call "AO SCTR Messenger.vi"("Notifier Name"=w441, "Actions"=AO_SCTR_Actions."Update and Run", "Offset (V)"=w445, "Amplitude (V)"=w444, "Samples Per Channel"=w443, "Start Delay (ms)"=w442) -> ()  [unwired: 9 in, 1 out]
                    }
                  }
                }
              }
              n382 = Bundle By Name(cluster=T17 {"Value"=0.0, "Parameter"=2049184} ("sCMOS Parameter"), "Value"=w405) -> (w416:T17)
              n383 = call "Orca Flash Messanger.vi"("Notifier Name"=w403, "Camera Actions"=Orca_Flash_Actions."SETPARAM", "sCMOS Parameter"=w416) -> ()  [unwired: 8 in, 5 out]
            }
            frame "Start Acquisition" {
              n384 = case shown="\"Capture\"" w458 {
                tunnel: w461 -> [_ w465 _]
                tunnel: [4Pi_Capture_Actions."Quit" ("y") 4Pi_Capture_Actions."Quit" ("y") 4Pi_Capture_Actions."Update SubFolder" ("y")] -> w460
                tunnel: w459 -> [_ _ w510]
                tunnel: w457 -> [_ _ w502]
                tunnel: w456 -> [w463 w466 w498]
                tunnel: [w463 w466 w497] -> w455
                tunnel: w454 -> [_ _ w493]
                tunnel: w453 -> [_ _ w471]
                frame Default {
                }
                frame "Live Preview" {
                  n385 = call "Orca Flash Messanger.vi"("Notifier Name"=w465, "Camera Actions"=Orca_Flash_Actions."PREVIEW") -> ()  [unwired: 9 in, 5 out]
                }
                frame "Capture" {
                  w474 = 4Pi_Dual_DM_-_Standard_Action."Read" ("Action")
                  w496 = sgl 0.0 ("Cycle")
                  n386 = Get Notifier Status(notifier=w493) -> (notifier out=w494:refnum<notifier>, current notification=w492:T7)  [unwired: 1 in, 3 out]
                  n387 = Bundle By Name(cluster=w492, "Capture?"=TRUE) -> (w491:T7)
                  n388 = call "Stages Messenger.vi"("Stage Notifier Name"=w502, "Actions"=Stage_Actions."Get Position") -> ("Positions"=w505:dbl[])  [unwired: 9 in, 4 out]
                  n389 = Send Notification(notification=w491, notifier=w494) -> ()  [unwired: 1 in, 2 out]
                  n390 = Index Array(array=w505, index=0) -> (element=w503:dbl)
                  n391 = call "4Pi Dual DM - Mirror Mode DUAL AE.vi"("Action"=w474) -> ("Mirror Modes Out"=w475:T35)  [unwired: 14 in]
                  n392 = call "4Pi Dual DM - Active Mirror AE.vi"("Action"=w474) -> ("Active Mirror"=w476:i32)  [unwired: 14 in]
                  n393 = call "Stages Messenger.vi"("Stage Notifier Name"=w471, "Actions"=Stage_Actions."SERVO ON/OFF", "Servo On?"=FALSE, "Exit While Busy?"=FALSE) -> ()  [unwired: 7 in, 5 out]
                  n394 = Index Array(array=w475, index (col)=w476) -> (element=w473:cluster{"Mode":string, "Amplitude":dbl}[])  [unwired: 1 in]
                  n395 = Get Notifier Status(notifier=w510) -> (notifier out=w507:refnum<notifier>, current notification=w508:T10)  [unwired: 1 in, 3 out]
                  n396 = Bundle By Name(cluster=w508, "Init Mirror Modes"=w473, "Init Z Position (µm)"=w503) -> (w499:T10)
                  n397 = Unbundle By Name(w499) -> ("No. Amp steps"=w478:u16, "No. Mirror Mode"=w477:u16, "Cycles"=w500:u16, "No. of Z Steps"=w501:u16)
                  n398 = Send Notification(notification=w499, notifier=w507) -> ()  [unwired: 1 in, 2 out]
                  n399 = local write "Z Step"(w496) -> ()
                  n400 = local write "Cycle"(w496) -> ()
                  n401 = local write "Frame"(u32 0 ("Frame")) -> ()
                  n402 = Bundle By Name(cluster=w498, "# of Amp steps"=w478, "# of Mirror Mode"=w477, "# of Cycles"=w500, "# of Steps"=w501) -> (w497:T22)
                  n403 = Obtain Notifier(name (unnamed)="WFDC External Sync", notification data type=T24 {"Cycle Sync"=enum."Pause Requested", "Z Offset"=0.0, "WFDC Status"=enum."Idle"} ("WFDC External Sync"), create if not found? (T)=FALSE) -> (notifier out=w480:refnum<notifier>, error out=w479:errorcluster)  [unwired: 1 in, 1 out]
                  n404 = Get Notifier Status(notifier=w480, error in (no error)=w479) -> (notifier out=w485:refnum<notifier>, current notification=w486:T24, error out=w487:errorcluster)  [unwired: 2 out]
                  n405 = Unbundle By Name(w486) -> ("WFDC Status"=w484:T23)
                  n406 = case shown="Default" w484 {
                    tunnel: w485 -> [w513 w518]
                    tunnel: w486 -> [_ w517]
                    tunnel: w487 -> [w512 w515]
                    tunnel: [w513 w516] -> w489
                    tunnel: [w512 w514] -> w488
                    frame Default {
                    }
                    frame "Error" {
                      n407 = Two Button Dialog(message="Reset Wide Field Drift Correction error?", 1:"No" ("F button name (\"Cancel\")"), 2:"Yes" ("T button name (\"OK\")")) -> (T button?=w522:bool)
                      n408 = case shown="True" w522 {
                        tunnel: w518 -> [w524 w529]
                        tunnel: w517 -> [_ w531]
                        tunnel: [w524 w527] -> w516
                        tunnel: w515 -> [w523 w526]
                        tunnel: [w523 w525] -> w514
                        frame False {
                        }
                        frame True {
                          n409 = Bundle By Name(cluster=w531, "WFDC Status"=WFDC_Status."Idle") -> (w528:T24)
                          n410 = Send Notification(notification=w528, notifier=w529, error in (no error)=w526) -> (notifier out=w527:refnum<notifier>, error out=w525:errorcluster)
                        }
                      }
                    }
                  }
                  n411 = case shown="Error" w488 {
                    tunnel: w489 -> [w511 _]
                    frame No Error {
                      n412 = Release Notifier(notifier=w511) -> ()  [unwired: 2 in, 3 out]
                    }
                    frame Error {
                    }
                  }
                }
              }
            }
            frame "Update SubFolder" {
              n413 = Equal?(x=w536, y=4Pi_Capture_Actions."Capture") -> (x = y?=w534:bool)
              n414 = And(x=w534, y="Auto Update Subfolder") -> (x .and. y?=w532:bool)
              n415 = case shown="True" w532 {
                tunnel: w538 -> [w545 w561]
                frame False {
                  n416 = Get Notifier Status(notifier=w545) -> (notifier out=w544:refnum<notifier>, current notification=w542:T10)  [unwired: 1 in, 3 out]
                  n417 = Unbundle By Name(w542) -> ("Base Path"=w541:path)
                  n418 = Bundle By Name(cluster=w542, "Save Path"=w541) -> (w543:T10)
                  n419 = Send Notification(notification=w543, notifier=w544) -> ()  [unwired: 1 in, 2 out]
                }
                frame True {
                  n420 = Get Notifier Status(notifier=w561) -> (notifier out=w549:refnum<notifier>, current notification=w548:T10)  [unwired: 1 in, 3 out]
                  n421 = feedback #1(u32 0) -> (w551:u32)
                  n422 = Unbundle By Name(w548) -> ("Base Path"=w560:path)
                  n423 = Increment(x=w551) -> (x+1=w550:u32)
                  n424 = feedback-in #1(w550) -> ()
                  n425 = Format Into String(format string="%03d", w550) -> (resulting string=w552:string)  [unwired: 2 in, 1 out]
                  n426 = Strip Path(path=w560) -> (stripped path=w559:path, name=w557:string)
                  n427 = Concatenate Strings("Subfolder Name", w552) -> (w555:string)
                  n428 = Build Path(base path=w559, name or relative path=w555) -> (appended path=w558:path)
                  n429 = Build Path(base path=w558, name or relative path=w557) -> (appended path=w547:path)
                  n430 = Bundle By Name(cluster=w548, "Save Path"=w547) -> (w546:T10)
                  n431 = Send Notification(notification=w546, notifier=w549) -> ()  [unwired: 1 in, 2 out]
                }
              }
            }
            frame "Write Metadata" {
              w569 = T5 0 items=["Idle", "Orthogonal", "Random"] ("y")
              w586 = T5 2 items=["Idle", "Orthogonal", "Random"] ("y")
              n432 = Get Notifier Status(notifier=w592) -> (notifier out=w589:refnum<notifier>, current notification=w572:T10)  [unwired: 1 in, 3 out]
              n433 = Not Equal?(x=4Pi_Capture_Actions."Capture", y=w591) -> (x != y?=w577:bool)
              n434 = Unbundle By Name(w572) -> ("Init Z Position (µm)"=w588:dbl, "Save Path"=w590:path, "Z Step Size (µm)"=w596:dbl, "No. of Z Steps"=w595:u16, "DM scan mode"=w587:T5)
              n435 = Equal?(x=w587, y=w586) -> (x = y?=w576:bool)
              n436 = Not(x=w576) -> (.not. x?=w575:bool)
              n437 = Less?(x=w595, y=u16 2) -> (x < y?=w593:bool)
              n438 = Equal To 0?(x=w596) -> (x = 0?=w594:bool)
              n439 = Compound Arithmetic op=OR(w594, w593, w577) -> (w578:bool)
              n440 = Compound Arithmetic op=OR(w575, w577) -> (w574:bool)
              n441 = Strip Path(path=w590) -> (stripped path=w582:path)  [unwired: 1 out]
              n442 = call <vilib>:"Check if File or Folder Exists.vi"("path"=w582) -> ("file or folder exists?"=w584:bool, "dup path"=w583:path)  [unwired: 8 in, 1 out]
              n443 = case shown="False" w584 {
                tunnel: [w621 w623] -> w573
                tunnel: w583 -> [w622 w623]
                frame False {
                  n444 = Create Folder(path (use dialog)=w622) -> (created path=w621:path)  [unwired: 2 in, 2 out]
                }
                frame True {
                }
              }
              n445 = case shown="False" w574 {
                tunnel: [w601 refnum<k0> refnum] -> w580
                tunnel: w573 -> [w600 _]
                frame False {
                  n446 = Build Path(base path=w600, name or relative path="DM Amplitude.txt") -> (appended path=w603:path)
                  n447 = Open/Create/Replace File(file path (use dialog)=w603, operation (0:open)=T31."replace or create") -> (refnum out=w601:refnum<file>)  [unwired: 4 in, 2 out]
                }
                frame True {
                }
              }
              n448 = case shown="False" w578 {
                tunnel: w588 -> [w617 _]
                tunnel: w573 -> [w607 _]
                tunnel: [w606 refnum<k0> refnum] -> w581
                frame False {
                  n449 = Build Path(base path=w607, name or relative path="Z Positions.txt") -> (appended path=w615:path)
                  n450 = Open/Create/Replace File(file path (use dialog)=w615, operation (0:open)=T31."replace or create") -> (refnum out=w612:refnum<file>, error out=w610:errorcluster)  [unwired: 4 in, 1 out]
                  n451 = Format Value(format string="%.4f\\n", value (0)=w617) -> (output string=w611:string)  [unwired: 1 in]
                  n452 = Write to Text File(file (use dialog)=w612, text=w611, error in=w610) -> (refnum out=w608:refnum<file>, error out=w609:errorcluster)  [unwired: 1 in, 1 out]
                  n453 = case shown="No Error" w609 {
                    tunnel: w608 -> [w618 _]
                    tunnel: [w618 refnum<k0> refnum] -> w606
                    frame No Error {
                    }
                    frame Error {
                    }
                  }
                }
                frame True {
                }
              }
              n454 = Build Array(w581, w580) -> (w579:refnum<file>[])
              n455 = Bundle By Name(cluster=w572, "Metadata File Ref"=w579) -> (w585:T10)
              n456 = local read "Soft trigger"() -> (w565:bool)
              n457 = local read "DM scan mode"() -> (w568:T5)
              n458 = Send Notification(notification=w585, notifier=w589) -> ()  [unwired: 1 in, 2 out]
              n459 = Select(t=4Pi_Capture_Actions."Setup", s=w565, f=4Pi_Capture_Actions."Write DM") -> (s? t:f=w562:T11)
              n460 = Equal?(x=w568, y=w569) -> (x = y?=w571:bool)
              n461 = Select(t=4Pi_Capture_Actions."Setup" ("y"), s=w571, f=w562) -> (s? t:f=w567:T11)
            }
            frame "Setup" {
              w630 = T5 0 items=["Idle", "Orthogonal", "Random"] ("y")
              # "Change lasers here"
              n462 = local read "DM scan mode"() -> (w631:T5)
              n463 = Not Equal?(x=w631, y=w630) -> (x != y?=w628:bool)
              n464 = And(x="Soft trigger", y=w628) -> (x .and. y?=w627:bool)
              n465 = Select(t=4Pi_Capture_Actions."Camera Soft Trigger" ("y"), s=w627, f=4Pi_Capture_Actions."Camera") -> (s? t:f=w624:T11)
            }
            frame "Camera" {
              w639 = T5 1 items=["Idle", "Orthogonal", "Random"] ("y")
              n466 = Get Notifier Status(notifier=w659) -> (notifier out=w666:refnum<notifier>, current notification=w654:T10)  [unwired: 1 in, 3 out]
              n467 = Unbundle By Name(w654) -> ("Save Path"=w662:path, "Frames"=w655:u32)
              n468 = local read "DM scan mode"() -> (w640:T5)
              n469 = Unbundle By Name(w652) -> ("Current Cycle"=w638:u16, "Current Step"=w637:u16, "Current Mirror Mode"=w636:u16, "Current Amp step"=w635:u16)
              n470 = Equal?(x=w640, y=w639) -> (x = y?=w634:bool)
              n471 = property on="Current Laser" class="Ring (strict)"() -> ("RingText.Text"=w653:string)  [unwired: 2 in, 2 out]
              n472 = call "4Pi Capture File Name Increment.vi"("Path In"=w662, "Laser Line"=w653, "Cycle"=w638, "Step"=w637, "Mirror Mode"=w636, "Amp step"=w635, "add DM"=w634) -> ("Path Out"=w663:path)  [unwired: 8 in]
              n473 = Get Notifier Status(notifier=w647) -> (notifier out=w651:refnum<notifier>, current notification=w650:T7)  [unwired: 1 in, 3 out]
              n474 = Bundle By Name(cluster=w650, "Camera Running?"=TRUE) -> (w648:T7)
              n475 = call "Orca Flash Messanger.vi"("Notifier Name"=w657, "Camera Actions"=Orca_Flash_Actions."Record Settings", "Path"=w663, "# of frames"=w655) -> ("Notifier Name Dup"=w665:string)  [unwired: 7 in, 4 out]
              n476 = call "Orca Flash Messanger.vi"("Notifier Name"=w665, "Camera Actions"=Orca_Flash_Actions."RECORD") -> ("Notifier Name Dup"=w660:string, "Image Ref"=w656:T6)  [unwired: 9 in, 3 out]
              n477 = Send Notification(notification=w648, notifier=w651) -> (notifier out=w646:refnum<notifier>)  [unwired: 1 in, 1 out]
              n478 = while {
                tunnel: w660 -> [w692]
                tunnel: [w689] -> w658
                tunnel: w666 -> [w679]
                tunnel: w656 -> [w678]
                tunnel: [w677] -> w642
                tunnel: w646 -> [w677]
                stop <- w685 stop-if-true
                n479 = Get Notifier Status(notifier=w679) -> (current notification=w691:T10)  [unwired: 1 in, 4 out]
                n480 = Unbundle By Name(w691) -> ("Running?"=w684:bool)
                n481 = Wait (ms)(milliseconds to wait=u32 10) -> ()  [unwired: 1 out]
                n482 = call "IMAQ Read Custom Data"("Key"="Image Data", "Image"=w678) -> ("Custom Data Out"=w675:string)  [unwired: 7 in, 2 out]
                n483 = Not(x=w684) -> (.not. x?=w688:bool)
                n484 = Unflatten From JSON(JSON string=w675, type and defaults=T32 {"Frame"=0, "Sensor Height"=0, "Sensor Width"=0, "ROI Height"=0, "ROI Width"=0, "ROI Enable?"=FALSE, "Bit per Pixel"=0} ("Camera IMAQ Key Info")) -> (value=w673:T32)  [unwired: 5 in, 1 out]
                n485 = Unbundle By Name(w673) -> ("Frame"=→"Frame" →"Current Frame":u32)
                n486 = Select(t=Orca_Flash_Actions."STATUS" ("Camera Actions"), s=w684, f=Orca_Flash_Actions."IDLE") -> (s? t:f=w680:T21)
                n487 = call "Orca Flash Messanger.vi"("Notifier Name"=w692, "Camera Actions"=w680) -> ("Running?"=w687:bool)  [unwired: 9 in, 4 out]
                n488 = Not(x=w687) -> (.not. x?=w686:bool)
                n489 = Or(x=w688, y=w686) -> (x .or. y?=w685:bool)
                n490 = Select(t=4Pi_Capture_Actions."Swtich1", s="DM first", f=4Pi_Capture_Actions."Switch" ("y")) -> (s? t:f=w668:T11)
                n491 = Select(t=w668, s=w684, f=4Pi_Capture_Actions."Abort") -> (s? t:f=w689:T11)
              }
              n492 = Get Notifier Status(notifier=w642) -> (notifier out=w641:refnum<notifier>, current notification=w643:T7)  [unwired: 1 in, 3 out]
              n493 = Bundle By Name(cluster=w643, "Camera Running?"=FALSE) -> (w645:T7)
              n494 = Send Notification(notification=w645, notifier=w641) -> ()  [unwired: 1 in, 2 out]
            }
            frame "Camera Soft Trigger" {
              n495 = Get Notifier Status(notifier=w726) -> (notifier out=w732:refnum<notifier>, current notification=w723:T10)  [unwired: 1 in, 3 out]
              n496 = Unbundle By Name(w723) -> ("Save Path"=w728:path, "Frames"=w707:u32, "Amp step size"=w704:dbl)
              n497 = Unbundle By Name(w701) -> ("Current Cycle"=w712:u16, "Current Step"=w711:u16, "Current Mirror Mode"=w705:u16, "Current Step"=w698:u16)
              n498 = property on="Current Laser" class="Ring (strict)"() -> ("RingText.Text"=w710:string)  [unwired: 2 in, 2 out]
              n499 = Equal To 0?(x=w698) -> (x = 0?=w697:bool)
              n500 = call "4Pi Capture File Name Increment.vi"("Path In"=w728, "Laser Line"=w710, "Cycle"=w712, "Step"=w711, "Mirror Mode"=w705, "Amp step"=u16 0, "add DM"=TRUE) -> ("Path Out"=w729:path)  [unwired: 8 in]
              n501 = Get Notifier Status(notifier=w718) -> (notifier out=w722:refnum<notifier>, current notification=w721:T7)  [unwired: 1 in, 3 out]
              n502 = Bundle By Name(cluster=w721, "Camera Running?"=TRUE) -> (w719:T7)
              n503 = call "Orca Flash Messanger.vi"("Notifier Name"=w725, "Camera Actions"=Orca_Flash_Actions."Record Settings", "Path"=w729, "# of frames"=w707) -> ("Notifier Name Dup"=w731:string)  [unwired: 7 in, 4 out]
              n504 = local read "Mirror Mode"() -> (w706:u16[])
              n505 = call "Orca Flash Messanger.vi"("Notifier Name"=w731, "Camera Actions"=Orca_Flash_Actions."SOFT TRIGGER") -> ("Notifier Name Dup"=w694:string, "Image Ref"=w724:T6)  [unwired: 9 in, 3 out]
              n506 = Send Notification(notification=w719, notifier=w722) -> (notifier out=w717:refnum<notifier>)  [unwired: 1 in, 1 out]
              n507 = Obtain Notifier(name (unnamed)=w694, notification data type=T33 {"Camera Actions"=enum."IDLE", "Received?"=FALSE, "Running?"=FALSE, "sCMOS Parameter"={"Value"=0.0, "Parameter"=0}, "sCMOS ROI"={"H Offset"=0, "V Offset"=0, "H Width"=0, "V Width"=0}, "Save Path"=path "", "# of frames"=0, "Image Ref"=refnum, "Trigger?"=FALSE} ("Camera Cluster")) -> (notifier out=w693:refnum<notifier>)  [unwired: 2 in, 2 out]
              n508 = while {
                tunnel: w732 -> [w757]
                tunnel: w724 -> [w753]
                tunnel: w717 -> [w741]
                tunnel: w707 -> [w751]
                tunnel: w706 -> [w756]
                tunnel: w705 -> [w755]
                tunnel: w704 -> [w754]
                tunnel: [w744] -> w703
                tunnel: [w743] -> w702
                tunnel: [w741] -> w699
                tunnel: w697 -> [w737]
                tunnel: [w736] -> w696
                tunnel: w693 -> [w734]
                i -> [w739]
                stop <- w749 stop-if-true
                n509 = Get Notifier Status(notifier=w757) -> (current notification=w759:T10)  [unwired: 1 in, 4 out]
                n510 = To Unsigned Long Integer(number=w739) -> (unsigned 32bit integer=w738:u32)
                n511 = Unbundle By Name(w759) -> ("Running?"=w748:bool)
                n512 = Increment(x=w738) -> (x+1=w740:u32)
                n513 = Greater Or Equal?(x=w740, y=w751) -> (x >= y?=w750:bool)
                n514 = flat-sequence {
                  tunnel: w751 -> [w768]
                  tunnel: w756 -> [w767]
                  tunnel: w755 -> [w766]
                  tunnel: w738 -> [w765]
                  tunnel: w754 -> [w764]
                  tunnel: w753 -> [w763]
                  tunnel: [w763] -> w752
                  tunnel: [w762] -> w742
                  tunnel: w738 -> [w762]
                  tunnel: w737 -> [w761]
                  tunnel: [w760] -> w735
                  tunnel: w734 -> [w760]
                  tunnel: w752 -> [w778]
                  tunnel: [w772] -> w743
                  tunnel: w742 -> [w771]
                  tunnel: [w770] -> w736
                  tunnel: w735 -> [w769]
                  frame #0 {
                    n515 = call "4Pi Capture Write DM.vi"("Next mode?"=w761, "Amp step size"=w764, "Current Amp Step"=w765, "Current Mirror Mode"=w766, "Mirror Mode"=w767, "No. Amp steps"=w768) -> ()  [unwired: 6 in]
                  }
                  frame #1 {
                    n516 = Get Notifier Status(notifier=w769) -> (notifier out=w777:refnum<notifier>, current notification=w776:T33)  [unwired: 1 in, 3 out]
                    n517 = Bundle By Name(cluster=w776, "Trigger?"=TRUE) -> (w774:T33)
                    n518 = Send Notification(notification=w774, notifier=w777) -> (notifier out=w770:refnum<notifier>, error out=w773:errorcluster)  [unwired: 1 in]
                    n519 = while {
                      tunnel: w778 -> [w790]
                      tunnel: w773 -> [w789]
                      tunnel: [w788] -> w772
                      tunnel: w771 -> [w786]
                      i -> [w780]
                      stop <- w779 stop-if-true
                      n520 = call "IMAQ Read Custom Data"("error in (no error)"=w789, "Key"="Image Data", "Image"=w790) -> ("Custom Data Out"=w792:string)  [unwired: 6 in, 2 out]
                      n521 = Unflatten From JSON(JSON string=w792, type and defaults=T32 {"Frame"=0, "Sensor Height"=0, "Sensor Width"=0, "ROI Height"=0, "ROI Width"=0, "ROI Enable?"=FALSE, "Bit per Pixel"=0} ("Camera IMAQ Key Info")) -> (value=w791:T32)  [unwired: 5 in, 1 out]
                      n522 = Unbundle By Name(w791) -> ("Frame"=w785:u32)
                      n523 = Wait (ms)(milliseconds to wait=u32 1) -> ()  [unwired: 1 out]
                      n524 = Greater Or Equal?(x=w780, y=1000) -> (x >= y?=w781:bool)
                      n525 = Decrement(x=w785) -> (x-1=w788:u32)
                      n526 = local write "Current Frame"(w785) -> ()
                      n527 = local write "Frame"(w785) -> ()
                      n528 = Equal?(x=w788, y=w786) -> (x = y?=w782:bool)
                      n529 = Or(x=w782, y=w781) -> (x .or. y?=w779:bool)
                    }
                  }
                }
                n530 = Not(x=w748) -> (.not. x?=w747:bool)
                n531 = Or(x=w747, y=w750) -> (x .or. y?=w749:bool)
                n532 = Wait (ms)(milliseconds to wait=u32 10) -> ()  [unwired: 1 out]
                n533 = Select(t=4Pi_Capture_Actions."Abort" ("f"), s=w747, f=4Pi_Capture_Actions."Switch") -> (s? t:f=w744:T11)
              }
              n534 = Release Notifier(notifier=w696) -> ()  [unwired: 2 in, 3 out]
              n535 = Get Notifier Status(notifier=w699) -> (notifier out=w713:refnum<notifier>, current notification=w714:T7)  [unwired: 1 in, 3 out]
              n536 = Bundle By Name(cluster=w714, "Camera Running?"=FALSE) -> (w716:T7)
              n537 = Bundle By Name(cluster=w701, "Current Amp step"=w702) -> (w700:T22)
              n538 = Send Notification(notification=w716, notifier=w713) -> ()  [unwired: 1 in, 2 out]
            }
            frame "Switch" {
              n539 = Get Notifier Status(notifier=w803) -> (current notification=w802:T10)  [unwired: 1 in, 4 out]
              n540 = Unbundle By Name(w802) -> ("Cycles"=w799:u16, "No. of Z Steps"=w800:u16)
              n541 = Bundle By Name(cluster=w801, "# of Cycles"=w799, "# of Steps"=w800) -> (w794:T22)
              n542 = Unbundle By Name(w794) -> ("Current Cycle"=w812:u16, "# of Cycles"=w811:u16, "Current Step"=w810:u16, "# of Steps"=w809:u16)
              n543 = Increment(x=w812) -> (x+1=w796:u16)
              n544 = Increment(x=w810) -> (x+1=w795:u16)
              n545 = To Single Precision Float(number=w796) -> (single precision float=w808:sgl)
              n546 = To Single Precision Float(number=w811) -> (single precision float=w807:sgl)
              n547 = To Single Precision Float(number=w795) -> (single precision float=w806:sgl)
              n548 = To Single Precision Float(number=w809) -> (single precision float=w805:sgl)
              n549 = Divide(x=w808, y=w807) -> (x/y=→"Cycle":sgl)
              n550 = Divide(x=w806, y=w805) -> (x/y=→"Z Step":sgl)
              n551 = call "4Pi Capture Scan Counter.vi"("Scan Tracker"=w794) -> ("Scan Tracker Out"=w822:T22, "Move stage?"=w815:bool, "F_MVR/T_MOV"=w819:bool, "Exit?"=w821:bool)  [unwired: 7 in]
              n552 = Select(t=4Pi_Capture_Actions."Cycle" ("y"), s=w819, f=4Pi_Capture_Actions."Step") -> (s? t:f=w816:T11)
              n553 = Select(t=w816, s=w815, f=4Pi_Capture_Actions."Setup") -> (s? t:f=w813:T11)
              n554 = Select(t=4Pi_Capture_Actions."Abort" ("y"), s=w821, f=w813) -> (s? t:f=w797:T11)
              n555 = case shown="\"Cycle\"" w797 {
                tunnel: w796 -> [_ w825 _]
                tunnel: w795 -> [_ _ w827]
                frame Default {
                }
                frame "Cycle" {
                  n556 = Increment(x=w825) -> (x+1=→"Current Cycle":u16)
                }
                frame "Step" {
                  n557 = Increment(x=w827) -> (x+1=→"Current Step":u16)
                }
              }
            }
            frame "Swtich1" {
              n558 = Unbundle By Name(w836) -> ("Current Cycle"=w848:u16, "# of Cycles"=w847:u16, "Current Step"=w846:u16, "# of Steps"=w845:u16)
              n559 = Increment(x=w848) -> (x+1=w840:u16)
              n560 = Increment(x=w846) -> (x+1=w839:u16)
              n561 = To Single Precision Float(number=w840) -> (single precision float=w844:sgl)
              n562 = To Single Precision Float(number=w847) -> (single precision float=w843:sgl)
              n563 = To Single Precision Float(number=w839) -> (single precision float=w842:sgl)
              n564 = To Single Precision Float(number=w845) -> (single precision float=w841:sgl)
              n565 = Divide(x=w844, y=w843) -> (x/y=w838:sgl)
              n566 = Divide(x=w842, y=w841) -> (x/y=w837:sgl)
              n567 = local write "Z Step"(w837) -> ()
              n568 = local write "Cycle"(w838) -> ()
              n569 = call "4Pi Capture Scan Counter 1.vi"("Scan Tracker"=w836) -> ("Scan Tracker Out"=w835:T22, "To cycle?"=w832:bool, "Move stage?"=w833:bool, "Exit?"=w834:bool)  [unwired: 7 in]
              n570 = Select(t=4Pi_Capture_Actions."Step" ("y"), s=w833, f=4Pi_Capture_Actions."Write DM") -> (s? t:f=w831:T11)
              n571 = Select(t=4Pi_Capture_Actions."Cycle" ("f"), s=w832, f=w831) -> (s? t:f=w849:T11)
              n572 = Select(t=4Pi_Capture_Actions."Abort" ("y"), s=w834, f=w849) -> (s? t:f=w829:T11)
              n573 = case shown="\"Cycle\"" w829 {
                tunnel: w840 -> [_ w854 _]
                tunnel: w839 -> [_ _ w856]
                frame Default {
                }
                frame "Cycle" {
                  n574 = Increment(x=w854) -> (x+1=w853:u16)
                  n575 = local write "Current Cycle"(w853) -> ()
                }
                frame "Step" {
                  n576 = Increment(x=w856) -> (x+1=w855:u16)
                  n577 = local write "Current Cycle"(w855) -> ()
                }
              }
            }
            frame "Step" {
              n578 = Get Notifier Status(notifier=w871) -> (current notification=w870:T10)  [unwired: 1 in, 4 out]
              n579 = Unbundle By Name(w870) -> ("Metadata File Ref"=w861:refnum<file>[], "Z Step Size (µm)"=w863:dbl, "No. of Z Steps"=w866:u16)
              n580 = Less?(x=w866, y=u16 2) -> (x < y?=w865:bool)
              n581 = Equal To 0?(x=w863) -> (x = 0?=w868:bool)
              n582 = Or(x=w868, y=w865) -> (x .or. y?=w867:bool)
              n583 = case shown="False" w867 {
                tunnel: w869 -> [w903 _]
                tunnel: w863 -> [w902 _]
                tunnel: w862 -> [w889 _]
                tunnel: w861 -> [w875 _]
                frame False {
                  # "Force the wait to happen before the position is read."
                  n584 = Unbundle By Name(w889) -> ("Current Step"=w888:u16)
                  n585 = Index Array(array=w875, index=0) -> (element=w873:refnum<file>)
                  n586 = Obtain Notifier(name (unnamed)="WFDC External Sync", notification data type=T24 {"Cycle Sync"=enum."Pause Requested", "Z Offset"=0.0, "WFDC Status"=enum."Idle"} ("WFDC External Sync"), create if not found? (T)=FALSE) -> (notifier out=w895:refnum<notifier>, error out=w901:errorcluster)  [unwired: 1 in, 1 out]
                  n587 = Get Notifier Status(notifier=w895, error in (no error)=w901) -> (notifier out=w890:refnum<notifier>, current notification=w887:T24, error out=w900:errorcluster)  [unwired: 2 out]
                  n588 = Unbundle By Name(w887) -> ("WFDC Status"=w896:T23)
                  n589 = Unbundle By Name(w900) -> ("status"=w899:bool)
                  n590 = Not Equal?(x=WFDC_Status."DC Active", y=w896) -> (x != y?=w898:bool)
                  n591 = Or(x=w898, y=w899) -> (x .or. y?=w891:bool)
                  n592 = case shown="False" w891 {
                    tunnel: w903 -> [w908 w925]
                    tunnel: w902 -> [w915 w924]
                    tunnel: w890 -> [w912 _]
                    tunnel: w888 -> [w917 _]
                    tunnel: w887 -> [w916 _]
                    tunnel: [u32 350 ("milliseconds to wait") u32 10 ("milliseconds to wait")] -> w886
                    tunnel: [w908 w918] -> w882
                    frame False {
                      n593 = To Double Precision Float(number=w917) -> (double precision float=w914:dbl)
                      n594 = Multiply(x=w915, y=w914) -> (x*y=w913:dbl)
                      n595 = Bundle By Name(cluster=w916, "Z Offset"=w913) -> (w911:T24)
                      n596 = Send Notification(notification=w911, notifier=w912) -> (notifier out=w909:refnum<notifier>)  [unwired: 1 in, 1 out]
                      n597 = Release Notifier(notifier=w909) -> ()  [unwired: 2 in, 3 out]
                    }
                    frame True {
                      n598 = Build Array(w924) -> (w923:dbl[])
                      n599 = call "Stages Messenger.vi"("Stage Notifier Name"=w925, "Actions"=Stage_Actions."MVR", "Setpoint"=w923, "Axis"=bool[] [TRUE], "Exit While Busy?"=FALSE) -> ("Stage Notifier Name (Dup)"=w918:string)  [unwired: 6 in, 4 out]
                    }
                  }
                  n600 = Wait (ms)(milliseconds to wait=w886) -> (millisecond timer value=w876:u32)
                  n601 = Set File Position(offset (in bytes) (0)=i64 0, refnum=w873, from (0:start)=enum16{"start", "end", "current"}."end") -> (refnum out=w879:refnum<file>, error out=w877:errorcluster)  [unwired: 1 in]
                  n602 = call "Stages Messenger.vi"("Stage Notifier Name"=w882, "Actions"=Stage_Actions."Get Position", "Velocity"=w876) -> ("Positions"=w884:dbl[])  [unwired: 8 in, 4 out]
                  n603 = Index Array(array=w884, index=0) -> (element=w878:dbl)
                  n604 = case shown="No Error" w877 {
                    tunnel: w879 -> [w905 _]
                    tunnel: w878 -> [w904 _]
                    frame No Error {
                      n605 = Format Value(format string="%.4f\\n", value (0)=w904) -> (output string=w907:string)  [unwired: 1 in]
                      n606 = Write to Text File(file (use dialog)=w905, text=w907) -> ()  [unwired: 2 in, 3 out]
                    }
                    frame Error {
                    }
                  }
                }
                frame True {
                }
              }
              n607 = local read "DM first"() -> (w860:bool)
              n608 = Select(t=4Pi_Capture_Actions."Write DM", s=w860, f=4Pi_Capture_Actions."Setup" ("y")) -> (s? t:f=w857:T11)
            }
            frame "Cycle" {
              w936 = T5 0 items=["Idle", "Orthogonal", "Random"] ("y")
              n609 = Unbundle By Name(w939) -> ("Current Cycle"=w938:u16)
              n610 = Get Notifier Status(notifier=w952) -> (current notification=w928:T10)  [unwired: 1 in, 4 out]
              n611 = Get Notifier Status(notifier=w943) -> (notifier out=w942:refnum<notifier>, current notification=w941:T7)  [unwired: 1 in, 3 out]
              n612 = Bundle By Name(cluster=w941, "Cycle Number"=w938) -> (w940:T7)
              n613 = Send Notification(notification=w940, notifier=w942) -> ()  [unwired: 1 in, 2 out]
              n614 = Unbundle By Name(w928) -> ("Init Z Position (µm)"=w944:dbl, "Z Step Size (µm)"=w948:dbl, "No. of Z Steps"=w947:u16)
              n615 = Unbundle By Name(w928) -> ("Sampling Time (s)"=w926:dbl)
              n616 = Equal To 0?(x=w948) -> (x = 0?=w951:bool)
              n617 = Less?(x=w947, y=u16 2) -> (x < y?=w950:bool)
              n618 = Or(x=w951, y=w950) -> (x .or. y?=w946:bool)
              n619 = Equal To 0?(x=w926) -> (x = 0?=w927:bool)
              n620 = case shown="False" w946 {
                tunnel: w945 -> [w958 _]
                tunnel: w944 -> [w960 _]
                frame False {
                  n621 = Obtain Notifier(name (unnamed)="WFDC External Sync", notification data type=T24 {"Cycle Sync"=enum."Pause Requested", "Z Offset"=0.0, "WFDC Status"=enum."Idle"} ("WFDC External Sync"), create if not found? (T)=FALSE) -> (notifier out=w966:refnum<notifier>, error out=w972:errorcluster)  [unwired: 1 in, 1 out]
                  n622 = Get Notifier Status(notifier=w966, error in (no error)=w972) -> (notifier out=w961:refnum<notifier>, current notification=w959:T24, error out=w971:errorcluster)  [unwired: 2 out]
                  n623 = Unbundle By Name(w959) -> ("WFDC Status"=w967:T23)
                  n624 = Unbundle By Name(w971) -> ("status"=w970:bool)
                  n625 = Not Equal?(x=WFDC_Status."DC Active", y=w967) -> (x != y?=w969:bool)
                  n626 = Or(x=w969, y=w970) -> (x .or. y?=w962:bool)
                  n627 = case shown="True" w962 {
                    tunnel: w961 -> [w976 _]
                    tunnel: w960 -> [_ w981]
                    tunnel: w959 -> [w975 _]
                    tunnel: w958 -> [_ w980]
                    tunnel: [u32 350 ("milliseconds to wait") u32 20 ("milliseconds to wait")] -> w957
                    frame False {
                      n628 = Bundle By Name(cluster=w975, "Z Offset"=0.0) -> (w978:T24)
                      n629 = Send Notification(notification=w978, notifier=w976) -> (notifier out=w977:refnum<notifier>)  [unwired: 1 in, 1 out]
                      n630 = Release Notifier(notifier=w977) -> ()  [unwired: 2 in, 3 out]
                    }
                    frame True {
                      n631 = Build Array(w981) -> (w982:dbl[])
                      n632 = call "Stages Messenger.vi"("Stage Notifier Name"=w980, "Actions"=Stage_Actions."MOVE", "Setpoint"=w982, "Axis"=bool[] [TRUE], "Exit While Busy?"=FALSE) -> ()  [unwired: 6 in, 5 out]
                    }
                  }
                  n633 = Wait (ms)(milliseconds to wait=w957) -> ()  [unwired: 1 out]
                }
                frame True {
                }
              }
              n634 = case shown="False" w927 {
                tunnel: w926 -> [w956 _]
                frame False {
                  n635 = Multiply(x=w956, y=1000.0) -> (x*y=w954:dbl)
                  n636 = Wait (ms)(milliseconds to wait=w954) -> ()  [unwired: 1 out]
                }
                frame True {
                }
              }
              n637 = local read "Soft trigger"() -> (w929:bool)
              n638 = local read "DM scan mode"() -> (w933:T5)
              n639 = Select(t=4Pi_Capture_Actions."External Cycle Sync" ("f"), s=w929, f=4Pi_Capture_Actions."Write DM") -> (s? t:f=w930:T11)
              n640 = Equal?(x=w933, y=w936) -> (x = y?=w935:bool)
              n641 = Select(t=4Pi_Capture_Actions."External Cycle Sync" ("y"), s=w935, f=w930) -> (s? t:f=w934:T11)
            }
            frame "Write DM" {
              n642 = Get Notifier Status(notifier=w1003) -> (current notification=w1002:T10)  [unwired: 1 in, 4 out]
              n643 = Unbundle By Name(w994) -> ("Current Mirror Mode"=w999:u16, "Current Amp step"=w1000:u16, "Current Step"=w986:u16)
              n644 = Unbundle By Name(w1002) -> ("DM scan mode"=w996:T5, "Amp step size"=w998:dbl, "No. Amp steps"=w997:u16, "Metadata File Ref"=w995:refnum<file>[])
              n645 = local read "Mirror Mode"() -> (w1001:u16[])
              n646 = case shown="1, Default" w996 {
                tunnel: [w1006 w1063] -> w1005
                tunnel: w1001 -> [w1011 w1059]
                tunnel: w1000 -> [_ w1046]
                tunnel: w999 -> [_ w1044]
                tunnel: w998 -> [_ w1051]
                tunnel: w997 -> [_ w1050]
                tunnel: w995 -> [w1010 _]
                tunnel: w986 -> [_ w1039]
                frame 2 {
                  w1012 = 4Pi_Dual_DM_-_Standard_Action."Read" ("Action")
                  n647 = Index Array(array=w1010, index=1) -> (element=w1008:refnum<file>)
                  n648 = Refnum to Path(1:w1008) -> (0:w1007:path)
                  n649 = call "4Pi Dual DM - Mirror Mode DUAL AE.vi"("Action"=w1012) -> ("Mirror Modes Out"=w1019:T35)  [unwired: 14 in]
                  n650 = call "4Pi Dual DM - Active Mirror AE.vi"("Action"=w1012) -> ("Active Mirror"=w1020:i32)  [unwired: 14 in]
                  n651 = Initialize Array(0.0 ("element"), 0 ("dimension size")) -> (w1016:dbl[])
                  n652 = Index Array(array=w1019, index (col)=w1020) -> (element=w1013:cluster{"Mode":string, "Amplitude":dbl}[])  [unwired: 1 in]
                  n653 = for {
                    tunnel: w1011 -> [w1026] mode=indexing
                    shift-right: [w1033] -> w1023
                    shift-left: w1016 -> [w1034]
                    tunnel: "Amp magnitude" -> [w1031]
                    shift-right: [w1028] -> w1018
                    shift-left: w1013 -> [w1029]
                    n654 = Decrement(x=w1026) -> (x-1=w1025:u16)
                    n655 = Multiply(x=w1031, y=2.0) -> (x*y=w1038:dbl)
                    n656 = Random Number (0-1)() -> (number: 0 to 1=w1036:dbl)
                    n657 = Multiply(x=w1036, y=w1038) -> (x*y=w1035:dbl)
                    n658 = Index Array(array=w1029, index=w1025) -> (element=w1032:cluster{"Mode":string, "Amplitude":dbl})
                    n659 = Subtract(x=w1035, y=w1031) -> (x-y=w1030:dbl)
                    n660 = Bundle By Name(cluster=w1032, "Amplitude"=w1030) -> (w1027:cluster{"Mode":string, "Amplitude":dbl})
                    n661 = Build Array (concatenate)(w1034, w1030) -> (w1033:dbl[])
                    n662 = Replace Array Subset(array=w1029, new element=w1027, index=w1025) -> (w1028:cluster{"Mode":string, "Amplitude":dbl}[])
                  }
                  n663 = Replace Array Subset(array=w1019, new element=w1018, index (col)=w1020) -> (w1006:T35)  [unwired: 1 in]
                  n664 = call-poly <vilib>:"Write Delimited Spreadsheet.vi"("file path (dialog if empty)"=w1007, "format (%.3f)"="%.4f", "1D data"=w1023, "append to file? (new file:F)"=TRUE, "delimiter (\\t)"="," ("delimiter (\\t)")) -> ()  [unwired: 9 in, 2 out]
                }
                frame 1, Default {
                  w1065 = 4Pi_Dual_DM_-_Standard_Action."Read" ("Action")
                  n665 = Equal To 0?(x=w1044) -> (x = 0?=w1045:bool)
                  n666 = Decrement(x=w1050) -> (x-1=w1049:u16)
                  n667 = case shown="True" w1045 {
                    tunnel: [w1067 w1068] -> w1058
                    tunnel: w1044 -> [w1066 w1068]
                    frame False {
                      n668 = Decrement(x=w1066) -> (x-1=w1067:u16)
                    }
                    frame True {
                    }
                  }
                  n669 = To Double Precision Float(number=w1049) -> (double precision float=w1048:dbl)
                  n670 = call "4Pi Dual DM - Mirror Mode DUAL AE.vi"("Action"=w1065) -> ("Mirror Modes Out"=w1064:T35)  [unwired: 14 in]
                  n671 = call "4Pi Dual DM - Active Mirror AE.vi"("Action"=w1065) -> ("Active Mirror"=w1060:i32)  [unwired: 14 in]
                  n672 = Divide(x=w1048, y=2.0) -> (x/y=w1053:dbl)
                  n673 = Index Array(array=w1059, index #1=w1058, index #2=w1044) -> (element #1=w1042:u16, element #2=w1041:u16)
                  n674 = Index Array(array=w1064, index (col)=w1060) -> (element=w1061:cluster{"Mode":string, "Amplitude":dbl}[])  [unwired: 1 in]
                  n675 = Multiply(x=w1051, y=w1053) -> (x*y=w1047:dbl)
                  n676 = Decrement(x=w1042) -> (x-1=w1043:u16)
                  n677 = Decrement(x=w1041) -> (x-1=w1040:u16)
                  n678 = Index Array(array=w1061, index #1=w1043, index #2=w1040) -> (element #1=w1056:cluster{"Mode":string, "Amplitude":dbl}, element #2=w1057:cluster{"Mode":string, "Amplitude":dbl})
                  n679 = case shown="0" w1046 {
                    tunnel: w1057 -> [w1082 w1094]
                    tunnel: w1051 -> [_ w1092]
                    tunnel: [w1080 w1090] -> w1054
                    tunnel: w1056 -> [w1078 w1089]
                    tunnel: [w1076 w1089] -> w1055
                    tunnel: w1047 -> [w1071 _]
                    tunnel: w1039 -> [w1075 _]
                    frame 0 {
                      n680 = Not Equal To 0?(x=w1075) -> (x != 0?=w1073:bool)
                      n681 = local read "DM first"() -> (w1074:bool)
                      n682 = Unbundle By Name(w1078) -> ("Amplitude"=w1079:dbl)
                      n683 = Unbundle By Name(w1082) -> ("Amplitude"=w1083:dbl)
                      n684 = Compound Arithmetic op=AND(w1074, w1073) -> (w1072:bool)
                      n685 = case shown="True" w1072 {
                        tunnel: w1071 -> [w1084 w1088]
                        tunnel: [w1084 w1086] -> w1070
                        tunnel: [w1084 0.0] -> w1069
                        frame False {
                        }
                        frame True {
                          n686 = Multiply(x=w1088, y=2.0) -> (x*y=w1086:dbl)
                        }
                      }
                      n687 = Subtract(x=w1079, y=w1069) -> (x-y=w1077:dbl)
                      n688 = Subtract(x=w1083, y=w1070) -> (x-y=w1081:dbl)
                      n689 = Bundle By Name(cluster=w1078, "Amplitude"=w1077) -> (w1076:cluster{"Mode":string, "Amplitude":dbl})
                      n690 = Bundle By Name(cluster=w1082, "Amplitude"=w1081) -> (w1080:cluster{"Mode":string, "Amplitude":dbl})
                    }
                    frame Default {
                      n691 = Unbundle By Name(w1094) -> ("Amplitude"=w1093:dbl)
                      n692 = Add(x=w1093, y=w1092) -> (x+y=w1091:dbl)
                      n693 = Bundle By Name(cluster=w1094, "Amplitude"=w1091) -> (w1090:cluster{"Mode":string, "Amplitude":dbl})
                    }
                  }
                  n694 = Replace Array Subset(array=w1061, new element #1=w1055, index #1=w1043, new element #2=w1054, index #2=w1040) -> (w1062:cluster{"Mode":string, "Amplitude":dbl}[])
                  n695 = Replace Array Subset(array=w1064, new element=w1062, index (col)=w1060) -> (w1063:T35)  [unwired: 1 in]
                }
              }
              n696 = Unbundle By Name(w994) -> ("Current Amp step"=w993:u16)
              n697 = local read "DM first"() -> (w992:bool)
              n698 = flat-sequence {
                tunnel: w1005 -> [w1095]
                frame #0 {
                  n699 = call "4Pi Dual DM - Mirror Mode DUAL AE.vi"("Action"=4Pi_Dual_DM_-_Standard_Action."Write", "Mirror Modes In"=w1095) -> ()  [unwired: 13 in, 1 out]
                }
                frame #1 {
                  w1097 = "Mirror Control Que" ("name (unnamed)")
                  n700 = Obtain Queue(max queue size (-1, unlimited)=10, name (unnamed)=w1097, element data type=w1097, create if not found? (T)=FALSE) -> (queue out=w1101:refnum<queue>, error out=w1100:errorcluster)  [unwired: 1 in, 1 out]
                  n701 = case shown="No Error" w1100 {
                    tunnel: w1101 -> [w1102 _]
                    frame No Error {
                      n702 = Enqueue Element(queue=w1102, element="Mirror Modes" ("name (unnamed)")) -> ()  [unwired: 2 in, 3 out]
                    }
                    frame Error {
                      n703 = One Button Dialog(message="DMs not found.") -> ()  [unwired: 1 in, 1 out]
                    }
                  }
                }
              }
              n704 = Not Equal To 0?(x=w993) -> (x != 0?=w991:bool)
              n705 = Compound Arithmetic op=AND(w992, w991) -> (w990:bool)
              n706 = Select(t=4Pi_Capture_Actions."Setup", s=w990, f=4Pi_Capture_Actions."External Cycle Sync" ("y")) -> (s? t:f=w987:T11)
            }
            frame "External Cycle Sync" {
              n707 = Obtain Notifier(name (unnamed)="WFDC External Sync", notification data type=T24 {"Cycle Sync"=enum."Pause Requested", "Z Offset"=0.0, "WFDC Status"=enum."Idle"} ("WFDC External Sync"), create if not found? (T)=FALSE) -> (notifier out=w1123:refnum<notifier>, error out=w1126:errorcluster)  [unwired: 1 in, 1 out]
              n708 = Get Notifier Status(notifier=w1123, error in (no error)=w1126) -> (notifier out=w1112:refnum<notifier>, current notification=w1111:T24, error out=w1125:errorcluster)  [unwired: 2 out]
              n709 = Unbundle By Name(w1125) -> ("status"=w1119:bool)
              n710 = Unbundle By Name(w1111) -> ("WFDC Status"=w1110:T23, "Cycle Sync"=w1118:T25)
              n711 = Not(x=w1119) -> (.not. x?=w1114:bool)
              n712 = Equal?(x=WFDC_Status."Error", y=w1110) -> (x = y?=w1108:bool)
              n713 = Equal?(x=WFDC_Status."DC Active", y=w1110) -> (x = y?=w1116:bool)
              n714 = Equal?(x=w1118, y=WFDC_Cycle_Pause."Pause Requested") -> (x = y?=w1115:bool)
              n715 = Compound Arithmetic op=AND(w1116, w1115, w1114) -> (w1113:bool)
              n716 = case shown="False" w1113 {
                tunnel: w1112 -> [_ w1136]
                tunnel: w1111 -> [_ w1138]
                frame False {
                }
                frame True {
                  n717 = Bundle By Name(cluster=w1138, "Cycle Sync"=WFDC_Cycle_Pause."Paused") -> (w1135:T24)
                  n718 = Send Notification(notification=w1135, notifier=w1136) -> (notifier out=w1134:refnum<notifier>)  [unwired: 1 in, 1 out]
                  n719 = while {
                    tunnel: w1134 -> [w1149]
                    tunnel: [w1140] -> w1131
                    tunnel: [w1139] -> w1133
                    i -> [w1145]
                    stop <- w1141 stop-if-true
                    n720 = Get Notifier Status(notifier=w1149) -> (notifier out=w1140:refnum<notifier>, current notification=w1139:T24)  [unwired: 1 in, 3 out]
                    n721 = Greater?(x=w1145, y=15000) -> (0:w1142:bool)
                    n722 = Unbundle By Name(w1139) -> ("Cycle Sync"=w1148:T25)
                    n723 = Equal?(x=w1148, y=WFDC_Cycle_Pause."Resume Requested") -> (x = y?=w1143:bool)
                    n724 = Or(x=w1143, y=w1142) -> (x .or. y?=w1141:bool)
                    n725 = Wait (ms)(milliseconds to wait=u32 1) -> ()  [unwired: 1 out]
                  }
                  n726 = Bundle By Name(cluster=w1133, "Cycle Sync"=WFDC_Cycle_Pause."Resumed") -> (w1130:T24)
                  n727 = Send Notification(notification=w1130, notifier=w1131) -> (notifier out=w1129:refnum<notifier>)  [unwired: 1 in, 1 out]
                  n728 = Release Notifier(notifier=w1129) -> ()  [unwired: 2 in, 3 out]
                }
              }
              n729 = Select(t=4Pi_Capture_Actions."Abort" ("y"), s=w1108, f=4Pi_Capture_Actions."Setup" ("y")) -> (s? t:f=w1106:T11)
            }
            frame "Quit" {
            }
          }
        }
      }
      n730 = local write "Quit"(w207) -> ()
      n731 = Release Notifier(notifier=w164) -> ()  [unwired: 2 in, 3 out]
    }
    frame Error {
      n732 = Release Notifier(notifier=w1561) -> (error out=w1560:errorcluster)  [unwired: 2 in, 2 out]
      n733 = for {
        tunnel: w1559 -> [w1566] mode=indexing
        n734 = call "IMAQ Dispose"("Image"=w1566) -> ()  [unwired: 5 in, 1 out]
      }
      n735 = Unbundle By Name(w1560) -> ("source"=w1563:string)
      n736 = Concatenate Strings("4Pi Capture Manager could not start.", "\r", w1563) -> (w1562:string)
      n737 = One Button Dialog(message=w1562) -> ()  [unwired: 1 in, 1 out]
    }
  }
  n738 = control-ref of="This VI"() -> (w100:refnum<vi>)
  n739 = property class="VI"(reference=w100) -> (reference out=w109:refnum<vi>, "Panel"=w101:refnum<vi>)  [unwired: 1 in, 1 out]
  n740 = property class="Pnl"(reference=w101) -> ("Decos[]"=w99:refnum<vi>[], "Panes[]"=w105:refnum<vi>[])  [unwired: 1 in, 2 out]
  n741 = Array Size(array=w99) -> (size(s)=w97:i32)
  n742 = Decrement(x=w97) -> (x-1=w98:i32)
  n743 = Index Array(array=w105, index=0) -> (element=w104:refnum<vi>)
  n744 = Index Array(array=w99, index=w98) -> (element=w107:refnum<vi>)
  n745 = property class="VI"(reference=w109) -> (reference out=w111:refnum<vi>, "Front Panel.PanelBounds"=w112:T36)  [unwired: 1 in, 1 out]
  n746 = property class="Decor"(reference=w107) -> ("Bounds"=w110:T37)  [unwired: 1 in, 2 out]
  n747 = property class="Pane"(reference=w104, "Origin"=T14 {"Horizontal"=0, "Vertical"=0}, "HorizScrollbarVisibility"=w108, "VertScrollbarVisibility"=w108) -> ()  [unwired: 1 in, 2 out]
  n748 = Unbundle By Name(w110) -> ("Width"=w115:u32, "Height"=w118:u32)
  n749 = control-ref of="Quit"() -> (w102:refnum<vi>)
  n750 = To Word Integer(number=w115) -> (16bit integer=w117:i16)
  n751 = To Word Integer(number=w118) -> ()  [unwired: 1 out]
  n752 = property class="Bool (strict)"(reference=w102) -> ("Height"=w120:u32, "Top"=w121:i32)  [unwired: 1 in, 2 out]
  n753 = Unbundle By Name(w112) -> ("Left"=w114:i16, "Top"=w125:i16)
  n754 = To Word Integer(number=w120) -> (16bit integer=w123:i16)
  n755 = To Word Integer(number=w121) -> (16bit integer=w124:i16)
  n756 = Add(x=w114, y=w117) -> (x+y=w116:i16)
  n757 = Compound Arithmetic op=ADD(w125, w123, w124, i16 12 ("y")) -> (w119:i16)
  n758 = Bundle By Name(cluster=w112, "Right"=w116, "Bottom"=w119) -> (w113:T36)
  n759 = property class="VI"(reference=w111, "Front Panel.PanelBounds"=w113) -> ()  [unwired: 1 in, 2 out]
